vi "Main.vi"() -> ()   [LabVIEW 2021]
uses:
  controls/SynchroCheckCentral.ctl
  controls/SynchroCheckCentral_Info.ctl
  controls/SynchroCheckCentral_Data.ctl
  controls/3ph Phasor.ctl
  controls/Phasor.ctl
  controls/AFE_froming_Central.ctl
  controls/AFE_froming_Central_Info.ctl
  controls/AFE_froming_Central_Data.ctl
  controls/references.ctl
  controls/Connected_OPF.ctl
  controls/Connected_OPF_Info.ctl
  controls/Connected_OPF_Data.ctl
  controls/Optimal_slack_selection.ctl
  controls/Optimal_slack_selection_Info.ctl
  controls/Optimal_slack_selection_Data.ctl
  controls/PVemulator_Central.ctl
  controls/PVemulator_Central_Info.ctl
  controls/PVemulator_Central_Data.ctl
  controls/measurements.ctl
  controls/measurements_SC.ctl
  controls/SC_references.ctl
  controls/MeteoBoxCentral.ctl
  controls/MeteoBoxCentral_Info.ctl
  controls/MeteoBoxCentral_Data.ctl
  controls/Setpoints_CDA.ctl
  controls/Setpoints_CDA_ZENONE.ctl
  controls/SCADA_to_SM.ctl
  controls/SCADAOGCentral_Info.ctl
  controls/SCADA_to_SM_Data.ctl
  controls/State Machine.ctl
  <vilib>/Platform/TimedLoop/XDataNode/timing_clust.ctl
  <vilib>/Platform/TimedLoop/XDataNode/nitl_modes.ctl
  <vilib>/Platform/TimedLoop/XDataNode/wakeup.ctl
  controls/PV_facade_central.ctl
  controls/PV_facade_cental_Info.ctl
  controls/PV_facade_central_Data.ctl
  <vilib>/JDP Science/JSONtext/Next JSON Value.vi
  <vilib>/JDP Science/JSONtext/String Subset.vi
  <vilib>/JDP Science/JSONtext/Parsing/Advance past next JSON Value (inlined COPY).vi
  <vilib>/JDP Science/JSONtext/Parsing/Advance past whitespace.vi
  <vilib>/JDP Science/JSONtext/Parsing/Advance past String.vi
  <vilib>/JDP Science/JSONtext/Parsing/Advance past Number.vi
  <vilib>/JDP Science/JSONtext/Parsing/Advance past Line Ending.vi
  <vilib>/JDP Science/JSONtext/Parsing/Parse Full Path or Item Name.vi
  <vilib>/JDP Science/JSONtext/Parsing/Advance past Array.vi
  <vilib>/JDP Science/JSONtext/Parsing/Advance past Object.vi
  <vilib>/JDP Science/JSONtext/support/Error Cluster From Code.vi
  <vilib>/JDP Science/JSONtext/Offset/Find Item Locations by Path.vi
  <vilib>/Utility/file.llb/Read Delimited Spreadsheet (DBL).vi
  <vilib>/Platform/TimedLoop/XDataNode/XDataNode.xnode
  <vilib>/Platform/TimedLoop/XDataNode/XDNodeRunTimeDep.lvlib
  <vilib>/JDP Science/JSONtext/JSONtext.lvlib
  <userlib>/_OpenG.lib/boolean/boolean.llb/openg_boolean__ogtk.lvlib
panel:
  out "V_afe":dbl
  out "V_upstream":dbl
  out "V_control":dbl
  out "V control":cluster{dbl, "ROCOF [Hz/s]":dbl}(graph)
  in  "PI on V":bool
  in  "SCADA":T1={"Info"={"Resource"="MeteoBox", "Problem"=FALSE, "Timestamp"=0.0}, "Data"={"Voltage mag"=[], "Voltage angle"=[]}}
  out "SCADA data":bool
  in  "OUT":T4
  in  "SC_include":bool
  out "time connected":timestamp
  out "time island":timestamp
  out "P_bess_island":dbl
  out "P_bess_connected":dbl
  out "P_pv_facade":dbl
  in  "SOC":dbl=40.0
  in  "bias magnitude":dbl
  in  "IN Meteo":T6={"Info"={"Resource"="MeteoBox", "Problem"=FALSE, "Timestamp"=0.0}, "Data"={"GI"=0.0, "GHI"=0.0, "GVI"=0.0, "Tair"=0.0, "Tcell roof"=0.0, "Global_Total_Irr"=0.0, "Diffused_Irr"=0.0, "Tcell facade"=0.0, "PV_mpp"={"perun"=0.0, "solarmax"=0.0, "facade"=0.0, "emul4"=0.0, "emul5"=0.0, "emul6"=0.0, "emul7"=0.0}}}
  out "SC_soc":dbl
  out "delta angle":dbl
  in  "Send sp DC?":bool
  in  "Send sp AC?":bool
  out "Zenone_Q":dbl
  out "Zenone_P":dbl
  out "forming SC?":bool
  out "OUT PV+SC":T9={"Info"={"Resource"="Zenone", "Problem"=FALSE, "Timestamp"=0.0}, "Data"={"Status 1"=FALSE, "Status 2"=FALSE, "measurements"={"V_PV1"=0.0, "V_CAP1"=0.0, "V_PV2"=0.0, "V_CAP2"=0.0, "V_grid2"=0.0, "V_PV3"=0.0, "V_CAP3"=0.0, "V_grid3"=0.0, "V_PV4"=0.0, "V_CAP4"=0.0, "V_grid4"=0.0, "V_grid1"=0.0, "P1"=0.0, "P2"=0.0, "P3"=0.0, "P4"=0.0}, "Status 3"=FALSE, "Status 4"=FALSE, "measurements SC"={"V_SC"=0.0, "V_CAP"=0.0, "V_grid"=0.0, "P"=0.0, "SOC"=0.0}, "Status SC"=FALSE, "Forming/Following"=FALSE, "Start forming"=FALSE, "SC references"={"Vdc"=0.0, "Pdc"=0.0}, "Start following"=FALSE}}
  out "PV data":bool
  out "AFE data":bool
  out "synchro data":bool
  in  "IN PV+SC":T9={"Info"={"Resource"="Zenone", "Problem"=FALSE, "Timestamp"=0.0}, "Data"={"Status 1"=FALSE, "Status 2"=FALSE, "measurements"={"V_PV1"=0.0, "V_CAP1"=0.0, "V_PV2"=0.0, "V_CAP2"=0.0, "V_grid2"=0.0, "V_PV3"=0.0, "V_CAP3"=0.0, "V_grid3"=0.0, "V_PV4"=0.0, "V_CAP4"=0.0, "V_grid4"=0.0, "V_grid1"=0.0, "P1"=0.0, "P2"=0.0, "P3"=0.0, "P4"=0.0}, "Status 3"=FALSE, "Status 4"=FALSE, "measurements SC"={"V_SC"=0.0, "V_CAP"=0.0, "V_grid"=0.0, "P"=0.0, "SOC"=0.0}, "Status SC"=FALSE, "Forming/Following"=FALSE, "Start forming"=FALSE, "SC references"={"Vdc"=0.0, "Pdc"=0.0}, "Start following"=FALSE}}
  out "iOPF data":bool
  out "cOPF data":bool
  in  "slack":T15={"Info"={"Resource"="Zenone", "Problem"=FALSE, "Timestamp"=0.0}, "Data"={"Operation mode"="Grid connected", "Optimal slack"="AFE 1", "Time-To-Live"=0.0}}
  in  "IN AFE":T18={"Info"={"Resource"="Zenone", "Problem"=FALSE, "Timestamp"=0.0}, "Data"={"Start forming 1"=FALSE, "Forming/Following"=[], "Start forming 2"=FALSE, "measurements"={"Vdc1"=0.0, "P1"=0.0, "Vdc2"=0.0, "P2"=0.0, "Q2"=0.0, "Vdc3"=0.0, "P3"=0.0, "Q3"=0.0, "Vdc4"=0.0, "P4"=0.0, "Q4"=0.0, "Q1"=0.0}, "Status"=[], "references"={"Vdc1"=0.0, "Vdc2"=0.0, "Qac2"=0.0, "Vdc3"=0.0, "Qac3"=0.0, "Vdc4"=0.0, "Qac4"=0.0, "Qac1"=0.0, "V_arg2"=0.0, "V_abs2"=0.0, "V_abs1"=0.0, "V_arg1"=0.0, "freq1"=0.0, "freq2"=0.0}, "Start following 1"=FALSE, "Start following 2"=FALSE}}
  in  "IN cOPF":T22={"Info"={"Resource"="Zenone", "Problem"=0.0, "Timestamp"=0.0}, "Data"={"Operation_mode"="Grid connected", "solution_feasible"=0.0, "Optimal_slack"="AFE 1", "setpoints"=[], "upper_layer_grid_info"={"Frequency"=0.0, "Angle"=0.0, "Magnitude"=0.0}, "SC_soc"=0.0, "PV"={"perun"=0.0, "solarmax"=0.0, "facade"=0.0, "emul4"=0.0, "emul5"=0.0, "emul6"=0.0, "emul7"=0.0}, "P_pv_facade"=0.0}}
  in  "IN iOPF":T22={"Info"={"Resource"="Zenone", "Problem"=0.0, "Timestamp"=0.0}, "Data"={"Operation_mode"="Grid connected", "solution_feasible"=0.0, "Optimal_slack"="AFE 1", "setpoints"=[], "upper_layer_grid_info"={"Frequency"=0.0, "Angle"=0.0, "Magnitude"=0.0}, "SC_soc"=0.0, "PV"={"perun"=0.0, "solarmax"=0.0, "facade"=0.0, "emul4"=0.0, "emul5"=0.0, "emul6"=0.0, "emul7"=0.0}, "P_pv_facade"=0.0}}
  in  "IN synchro":T25={"Info"={"Resource"="SyncroCheck", "Problem"=FALSE, "Timestamp"=0.0}, "Data"={"close/open relay"=TRUE, "Operation mode"="Grid connected", "V_Downstream"={"Phase A"={"Frequency"=0.0, "Magnitude"=0.0, "Angle [Deg]"=0.0}, "Phase B"={"Frequency"=0.0, "Magnitude"=0.0, "Angle [Deg]"=0.0}, "Phase C"={"Frequency"=0.0, "Magnitude"=0.0, "Angle [Deg]"=0.0}, "Phase N"={"Frequency"=0.0, "Magnitude"=0.0, "Angle [Deg]"=0.0}}, "V_UpStream"={"Phase A"={"Frequency"=0.0, "Magnitude"=0.0, "Angle [Deg]"=0.0}, "Phase B"={"Frequency"=0.0, "Magnitude"=0.0, "Angle [Deg]"=0.0}, "Phase C"={"Frequency"=0.0, "Magnitude"=0.0, "Angle [Deg]"=0.0}, "Phase N"={"Frequency"=0.0, "Magnitude"=0.0, "Angle [Deg]"=0.0}}, "Synchronised?"=TRUE}}
  out "OUT iOPF":T22={"Info"={"Resource"="Zenone", "Problem"=0.0, "Timestamp"=0.0}, "Data"={"Operation_mode"="Grid connected", "solution_feasible"=0.0, "Optimal_slack"="AFE 1", "setpoints"=[], "upper_layer_grid_info"={"Frequency"=0.0, "Angle"=0.0, "Magnitude"=0.0}, "SC_soc"=0.0, "PV"={"perun"=0.0, "solarmax"=0.0, "facade"=0.0, "emul4"=0.0, "emul5"=0.0, "emul6"=0.0, "emul7"=0.0}, "P_pv_facade"=0.0}}
  out "OUT cOPF":T22={"Info"={"Resource"="Zenone", "Problem"=0.0, "Timestamp"=0.0}, "Data"={"Operation_mode"="Grid connected", "solution_feasible"=0.0, "Optimal_slack"="AFE 1", "setpoints"=[], "upper_layer_grid_info"={"Frequency"=0.0, "Angle"=0.0, "Magnitude"=0.0}, "SC_soc"=0.0, "PV"={"perun"=0.0, "solarmax"=0.0, "facade"=0.0, "emul4"=0.0, "emul5"=0.0, "emul6"=0.0, "emul7"=0.0}, "P_pv_facade"=0.0}}
  out "OUT AFE":T18={"Info"={"Resource"="Zenone", "Problem"=FALSE, "Timestamp"=0.0}, "Data"={"Start forming 1"=FALSE, "Forming/Following"=[], "Start forming 2"=FALSE, "measurements"={"Vdc1"=0.0, "P1"=0.0, "Vdc2"=0.0, "P2"=0.0, "Q2"=0.0, "Vdc3"=0.0, "P3"=0.0, "Q3"=0.0, "Vdc4"=0.0, "P4"=0.0, "Q4"=0.0, "Q1"=0.0}, "Status"=[], "references"={"Vdc1"=0.0, "Vdc2"=0.0, "Qac2"=0.0, "Vdc3"=0.0, "Qac3"=0.0, "Vdc4"=0.0, "Qac4"=0.0, "Qac1"=0.0, "V_arg2"=0.0, "V_abs2"=0.0, "V_abs1"=0.0, "V_arg1"=0.0, "freq1"=0.0, "freq2"=0.0}, "Start following 1"=FALSE, "Start following 2"=FALSE}}
  out "OUT Synchro":T25={"Info"={"Resource"="SyncroCheck", "Problem"=FALSE, "Timestamp"=0.0}, "Data"={"close/open relay"=TRUE, "Operation mode"="Grid connected", "V_Downstream"={"Phase A"={"Frequency"=0.0, "Magnitude"=0.0, "Angle [Deg]"=0.0}, "Phase B"={"Frequency"=0.0, "Magnitude"=0.0, "Angle [Deg]"=0.0}, "Phase C"={"Frequency"=0.0, "Magnitude"=0.0, "Angle [Deg]"=0.0}, "Phase N"={"Frequency"=0.0, "Magnitude"=0.0, "Angle [Deg]"=0.0}}, "V_UpStream"={"Phase A"={"Frequency"=0.0, "Magnitude"=0.0, "Angle [Deg]"=0.0}, "Phase B"={"Frequency"=0.0, "Magnitude"=0.0, "Angle [Deg]"=0.0}, "Phase C"={"Frequency"=0.0, "Magnitude"=0.0, "Angle [Deg]"=0.0}, "Phase N"={"Frequency"=0.0, "Magnitude"=0.0, "Angle [Deg]"=0.0}}, "Synchronised?"=TRUE}}
  out "Time-To-Live (minutes)":dbl=134.0
  out "setpoints":dbl[](array[numeric])
  in  "nb instances":i16=7
  out "optimal_slack":string(combo)="AFE 1"
  out "iOPF valid":bool
  out "forming AFE?":bool
  out "cOPF valid?":bool
  out "synchronised?":bool
  in  "to grid connection":bool
  in  "to prepare for grid connection":bool
  in  "to island":bool
  in  "Stop":bool
  in  "to prepare for island":bool
  # "Islanding Manoeuvre - State Machine"
  # "synchronised"
  # "opf connected OK"
  # "opf island OK"
  # "forming AFE?"
  # "forming SC?"
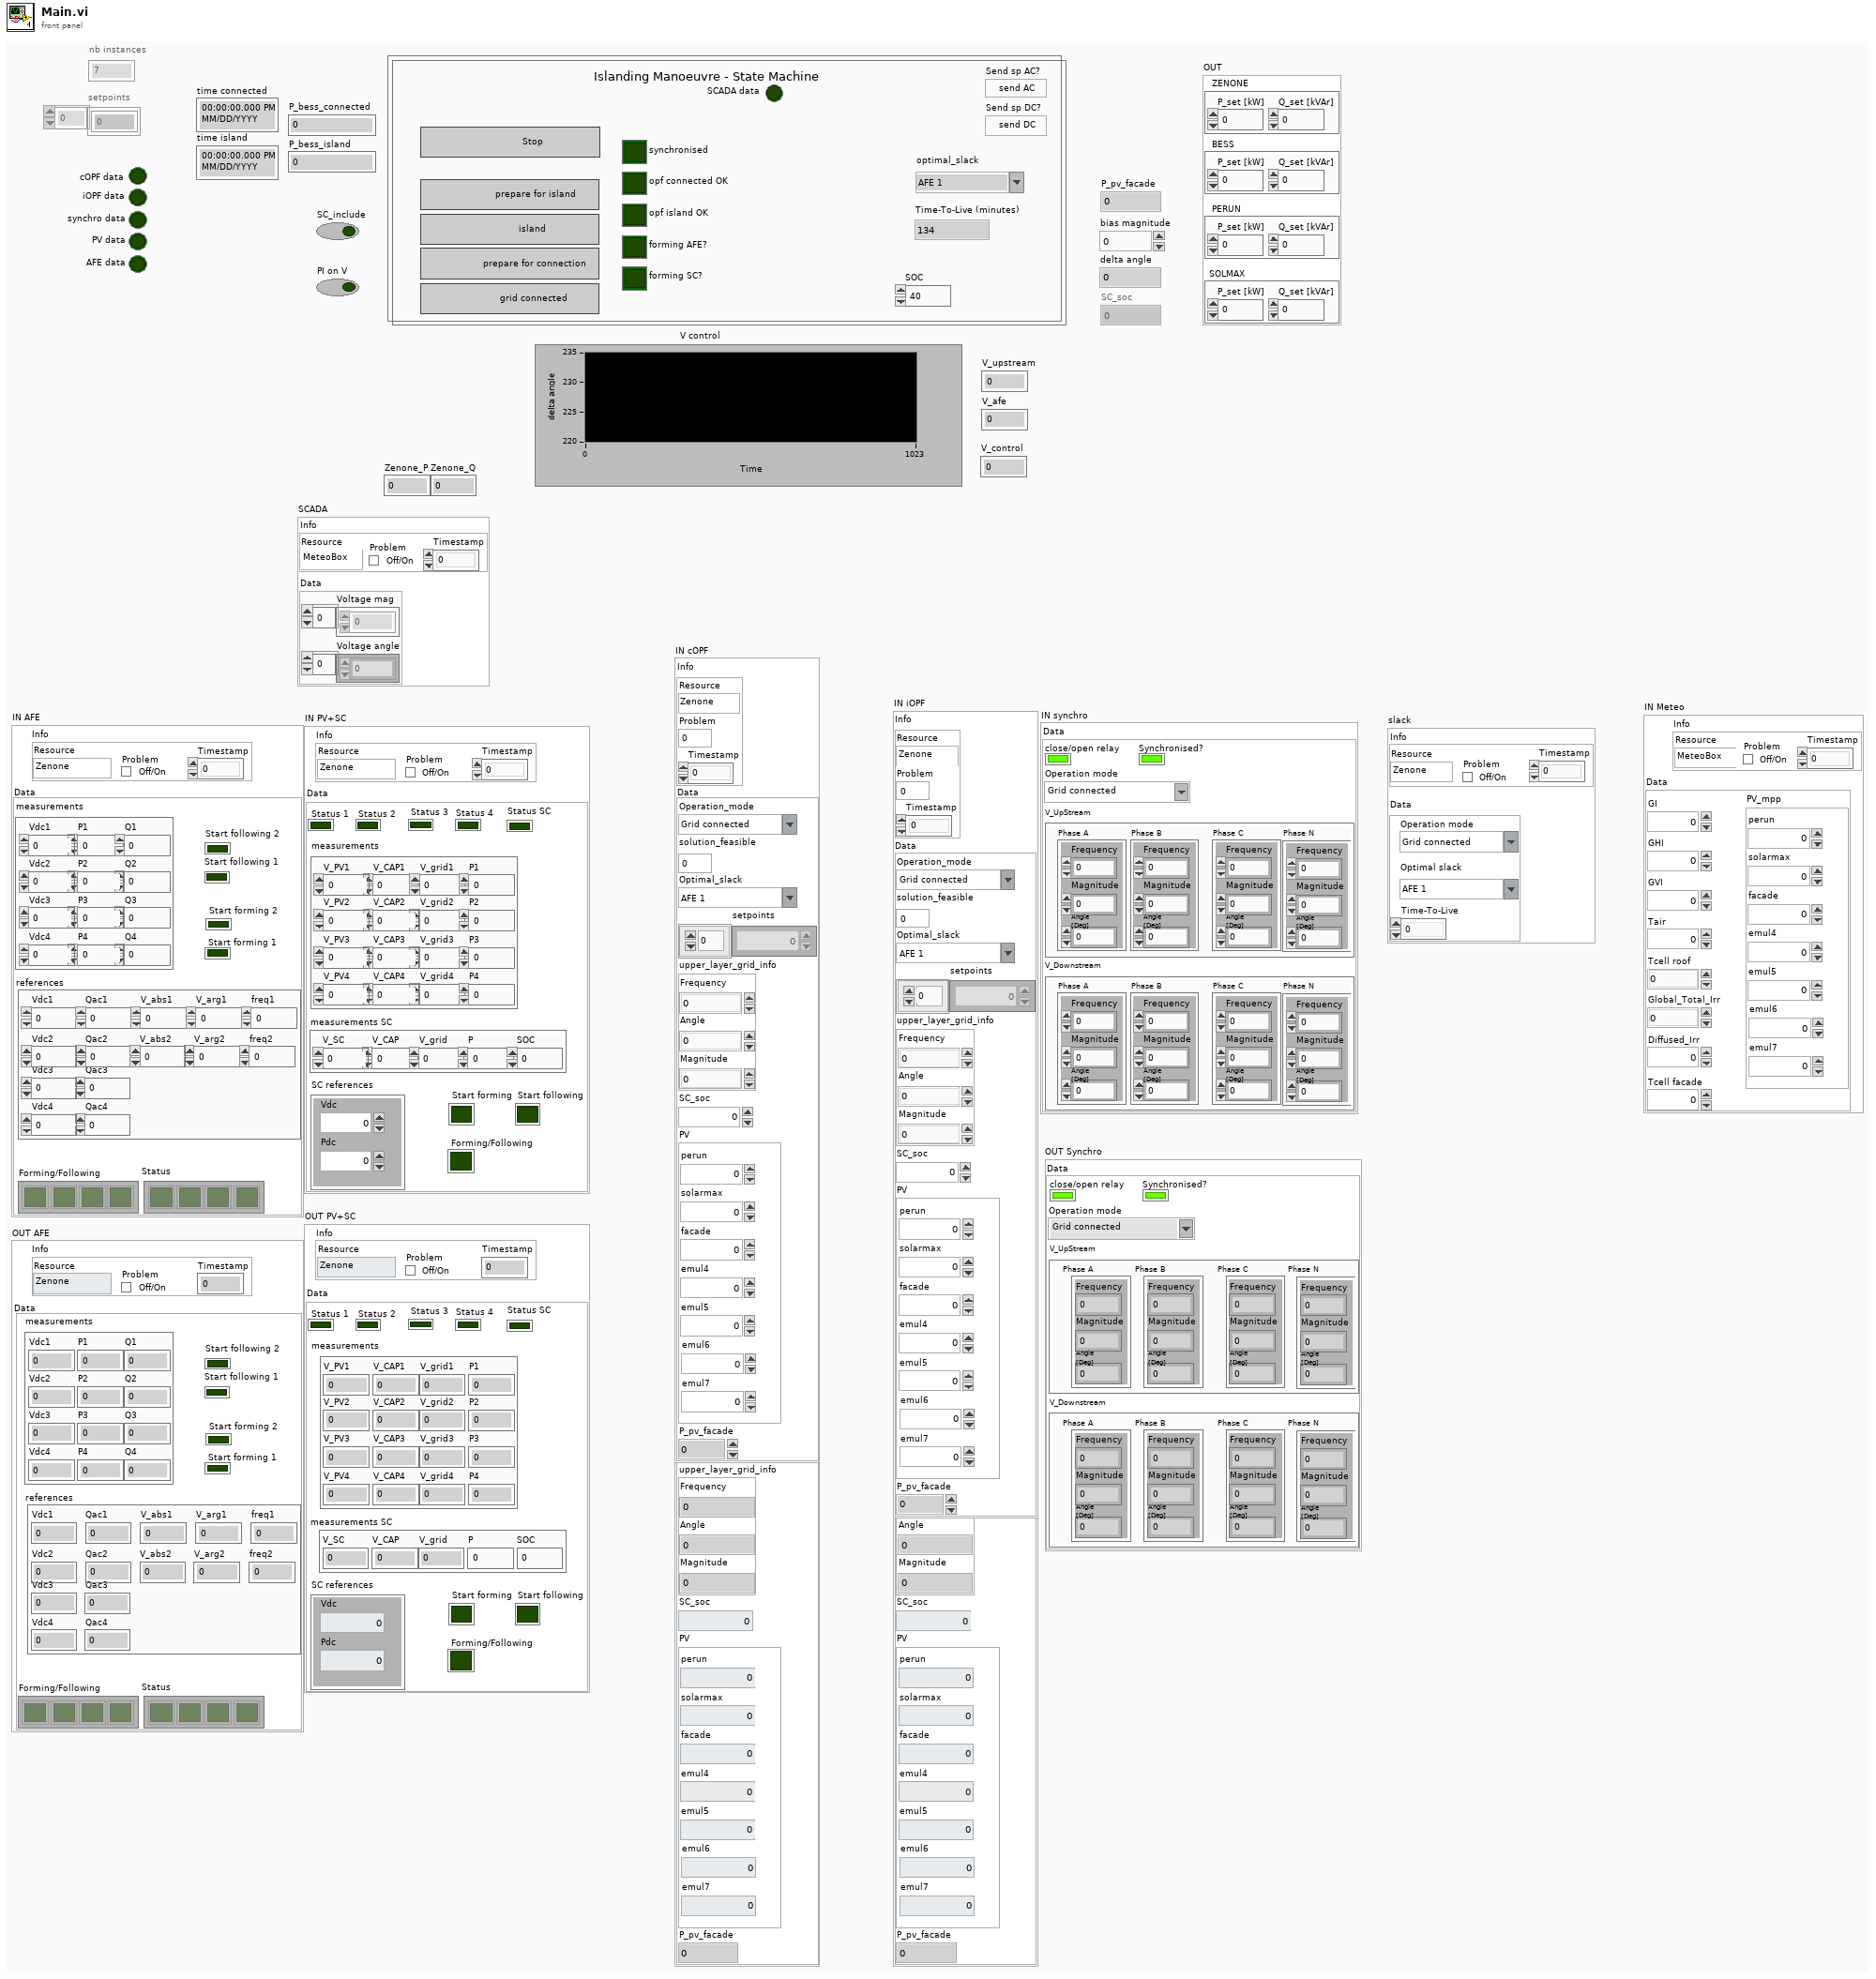
[diagram p1: front panel]
types:
  T1 = typedef "SCADA_to_SM.ctl" = cluster{"Info":T2, "Data":T3}
  T2 = typedef "SCADAOGCentral_Info.ctl" = cluster{"Resource":string, "Problem":bool, "Timestamp":dbl}
  T3 = typedef "SCADA_to_SM_Data.ctl" = cluster{"Voltage mag":dbl[], "Voltage angle":dbl[]}
  T4 = typedef "Setpoints_CDA.ctl" = cluster{"ZENONE":T5, "BESS":T5, "PERUN":T5, "SOLMAX":T5}
  T5 = typedef "Setpoints_CDA_ZENONE.ctl" = cluster{"P_set [kW]":dbl, "Q_set [kVAr]":dbl}
  T6 = typedef "MeteoBoxCentral.ctl" = cluster{"Info":T7, "Data":T8}
  T7 = typedef "MeteoBoxCentral_Info.ctl" = cluster{"Resource":string, "Problem":bool, "Timestamp":dbl}
  T8 = typedef "MeteoBoxCentral_Data.ctl" = cluster{"GI":dbl, "GHI":dbl, "GVI":dbl, "Tair":dbl, "Tcell roof":dbl, "Global_Total_Irr":dbl, "Diffused_Irr":dbl, "Tcell facade":dbl, "PV_mpp":cluster{"perun":dbl, "solarmax":dbl, "facade":dbl, "emul4":dbl, "emul5":dbl, "emul6":dbl, "emul7":dbl}}
  T9 = typedef "PVemulator_Central.ctl" = cluster{"Info":T10, "Data":T11}
  T10 = typedef "PVemulator_Central_Info.ctl" = cluster{"Resource":string, "Problem":bool, "Timestamp":dbl}
  T11 = typedef "PVemulator_Central_Data.ctl" = cluster{"Status 1":bool, "Status 2":bool, "measurements":T12, "Status 3":bool, "Status 4":bool, "measurements SC":T13, "Status SC":bool, "Forming/Following":bool, "Start forming":bool, "SC references":T14, "Start following":bool}
  T12 = typedef "measurements.ctl" = cluster{"V_PV1":dbl, "V_CAP1":dbl, "V_PV2":dbl, "V_CAP2":dbl, "V_grid2":dbl, "V_PV3":dbl, "V_CAP3":dbl, "V_grid3":dbl, "V_PV4":dbl, "V_CAP4":dbl, "V_grid4":dbl, "V_grid1":dbl, "P1":dbl, "P2":dbl, "P3":dbl, "P4":dbl}
  T13 = typedef "measurements_SC.ctl" = cluster{"V_SC":dbl, "V_CAP":dbl, "V_grid":dbl, "P":dbl, "SOC":dbl}
  T14 = typedef "SC_references.ctl" = cluster{"Vdc":dbl, "Pdc":dbl}
  T15 = typedef "Optimal_slack_selection.ctl" = cluster{"Info":T16, "Data":T17}
  T16 = typedef "Optimal_slack_selection_Info.ctl" = cluster{"Resource":string, "Problem":bool, "Timestamp":dbl}
  T17 = typedef "Optimal_slack_selection_Data.ctl" = cluster{"Operation mode":string, "Optimal slack":string, "Time-To-Live":dbl}
  T18 = typedef "AFE_froming_Central.ctl" = cluster{"Info":T19, "Data":T20}
  T19 = typedef "AFE_froming_Central_Info.ctl" = cluster{"Resource":string, "Problem":bool, "Timestamp":dbl}
  T20 = typedef "AFE_froming_Central_Data.ctl" = cluster{"Start forming 1":bool, "Forming/Following":bool[], "Start forming 2":bool, "measurements":cluster{"Vdc1":dbl, "P1":dbl, "Vdc2":dbl, "P2":dbl, "Q2":dbl, "Vdc3":dbl, "P3":dbl, "Q3":dbl, "Vdc4":dbl, "P4":dbl, "Q4":dbl, "Q1":dbl}, "Status":bool[], "references":T21, "Start following 1":bool, "Start following 2":bool}
  T21 = typedef "references.ctl" = cluster{"Vdc1":dbl, "Vdc2":dbl, "Qac2":dbl, "Vdc3":dbl, "Qac3":dbl, "Vdc4":dbl, "Qac4":dbl, "Qac1":dbl, "V_arg2":dbl, "V_abs2":dbl, "V_abs1":dbl, "V_arg1":dbl, "freq1":dbl, "freq2":dbl}
  T22 = typedef "Connected_OPF.ctl" = cluster{"Info":T23, "Data":T24}
  T23 = typedef "Connected_OPF_Info.ctl" = cluster{"Resource":string, "Problem":dbl, "Timestamp":dbl}
  T24 = typedef "Connected_OPF_Data.ctl" = cluster{"Operation_mode":string, "solution_feasible":dbl, "Optimal_slack":string, "setpoints":dbl[], "upper_layer_grid_info":cluster{"Frequency":dbl, "Angle":dbl, "Magnitude":dbl}, "SC_soc":dbl, "PV":cluster{"perun":dbl, "solarmax":dbl, "facade":dbl, "emul4":dbl, "emul5":dbl, "emul6":dbl, "emul7":dbl}, "P_pv_facade":dbl}
  T25 = typedef "SynchroCheckCentral.ctl" = cluster{"Info":T26, "Data":T27}
  T26 = typedef "SynchroCheckCentral_Info.ctl" = cluster{"Resource":string, "Problem":bool, "Timestamp":dbl}
  T27 = typedef "SynchroCheckCentral_Data.ctl" = cluster{"close/open relay":bool, "Operation mode":string, "V_Downstream":T28, "V_UpStream":T28, "Synchronised?":bool}
  T28 = typedef "3ph Phasor.ctl" = cluster{"Phase A":T29, "Phase B":T29, "Phase C":T29, "Phase N":T29}
  T29 = typedef "Phasor.ctl" = cluster{"Frequency":dbl, "Magnitude":dbl, "Angle [Deg]":dbl}
  T30 = typedef "State Machine.ctl" = enum16{"Grid connected", "Prepare for island", "Forming but connected", "Island", "Prepare for connection"}
  T31 = typedef "PV_facade_central.ctl" = cluster{"Info":T32, "Data":T33}
  T32 = typedef "PV_facade_cental_Info.ctl" = cluster{"Resource":string, "Problem":bool, "Timestamp":dbl}
  T33 = typedef "PV_facade_central_Data.ctl" = cluster{"P":dbl, "Q":dbl, "Pset":dbl, "Qset":dbl}
  T34 = typedef "XDNodeRunTimeDep.lvlib/timing_clust.ctl" = cluster{"Expected End [f-1]":u64, "Actual End [f-1]":u64, "Finished Late? [f-1]":bool, "Expected End [i-1]":u64, "Actual End [i-1]":u64, "Finished Late? [i-1]":bool, "Expected Start [i]":u64, "Actual Start [i]":u64, "Expected Start [f]":u64, "Actual Start [f]":u64, "Source Name":string, "Structure Name":string, "Period":i64, "Deadline":i64, "Offset":i64, "Start":i64, "Priority":i32, "Timeout":i32, "Mode":T35, "Wakeup Reason":T36, "Error":errorcluster, "Source Type":string, "Secondary Source Type":string, "Global End Time":u64, "Global Start Time":u64, "Frame Duration":u64, "Iteration Duration":u64, "Assigned CPU":i32, "I/O Scan Engine Mode":u32}
  T35 = typedef "XDNodeRunTimeDep.lvlib/nitl_modes.ctl" = enum32{"No Change", "Process missed periods, maintain original phase", "Discard missed periods, maintain original phase", "Process missed periods, ignore original phase", "Discard missed periods, ignore original phase"}
  T36 = typedef "XDNodeRunTimeDep.lvlib/wakeup.ctl" = enum32{"Normal", "Aborted", "Asynchronous wakeup", "Timing source error", "Timed loop error", "Timeout"}
  T37 = cluster{"Frequency":dbl, "Angle":dbl, "Magnitude":dbl}
  T38 = cluster{"perun":dbl, "solarmax":dbl, "facade":dbl, "emul4":dbl, "emul5":dbl, "emul6":dbl, "emul7":dbl}
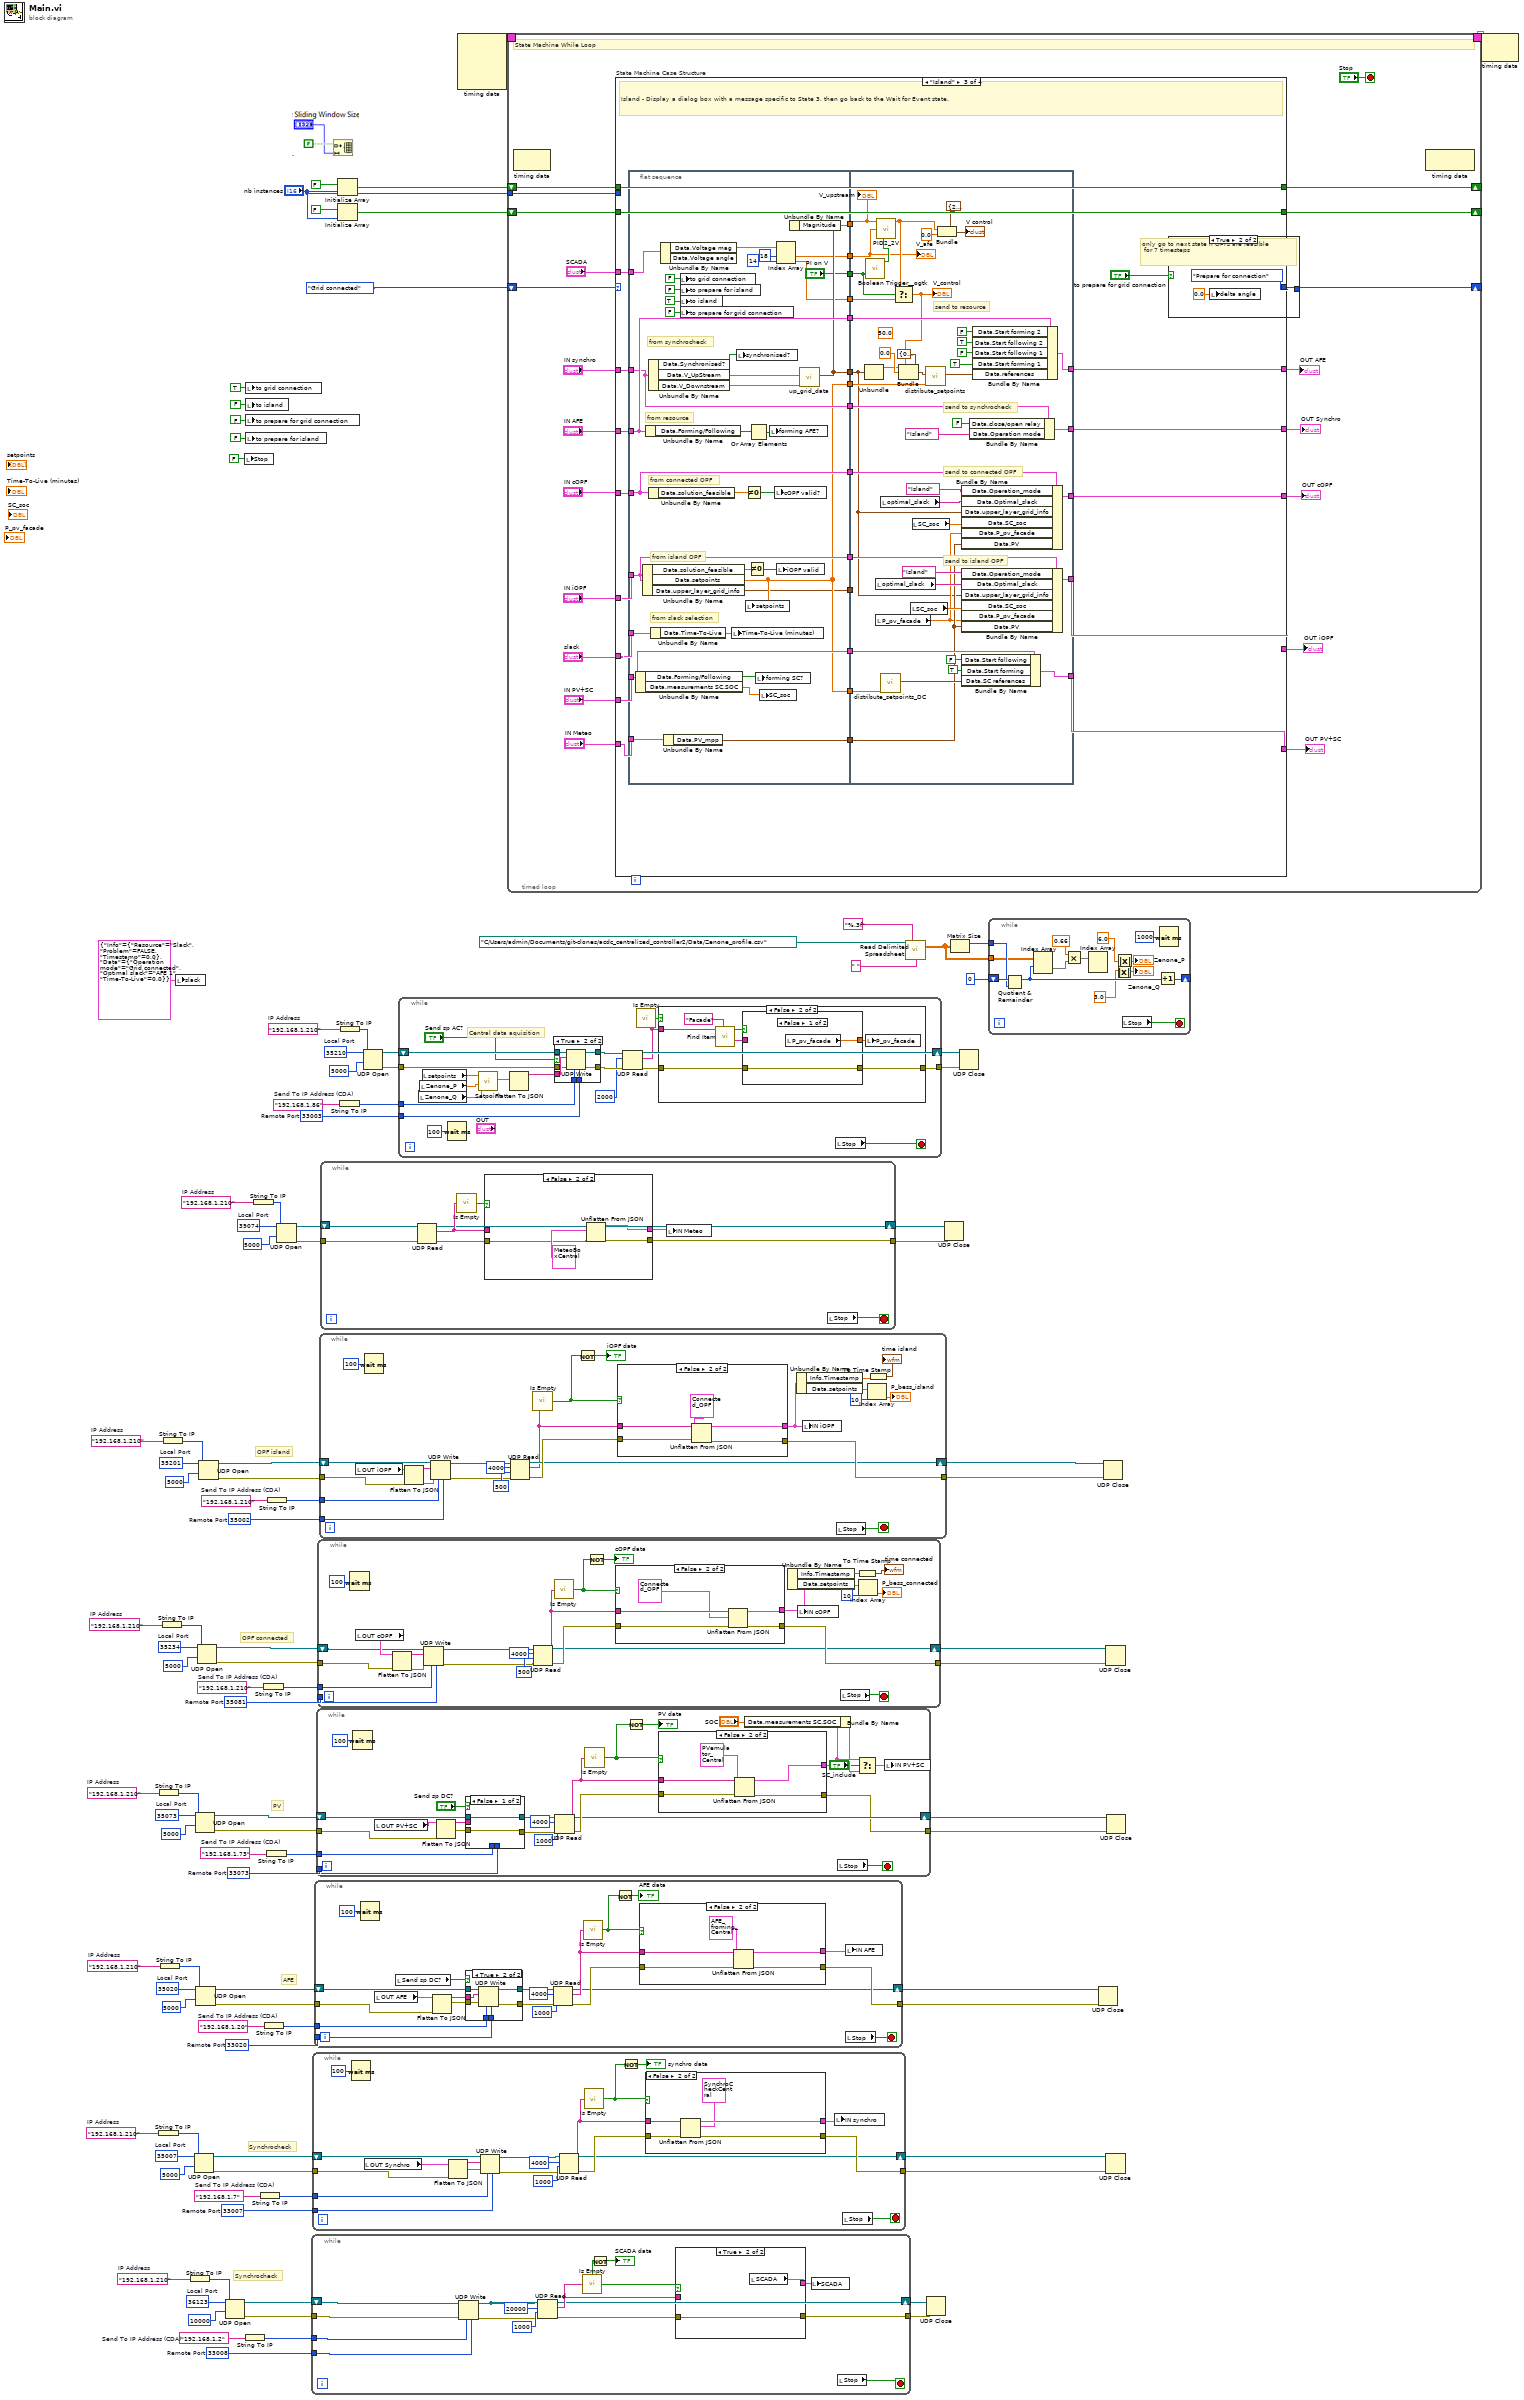
[diagram p0: block diagram]
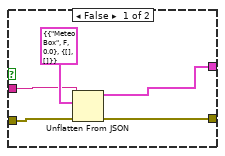
[diagram p2: hidden frame]
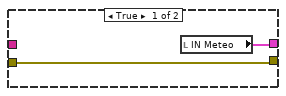
[diagram p3: hidden frame]
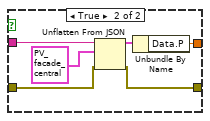
[diagram p5: hidden frame]
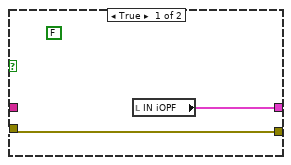
[diagram p7: hidden frame]
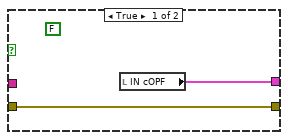
[diagram p8: hidden frame]
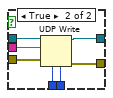
[diagram p9: hidden frame]
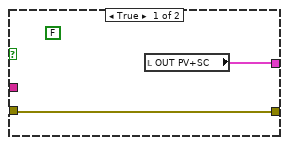
[diagram p10: hidden frame]
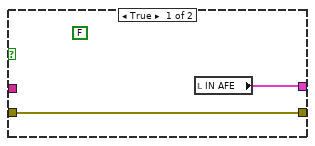
[diagram p12: hidden frame]
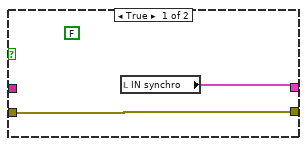
[diagram p13: hidden frame]
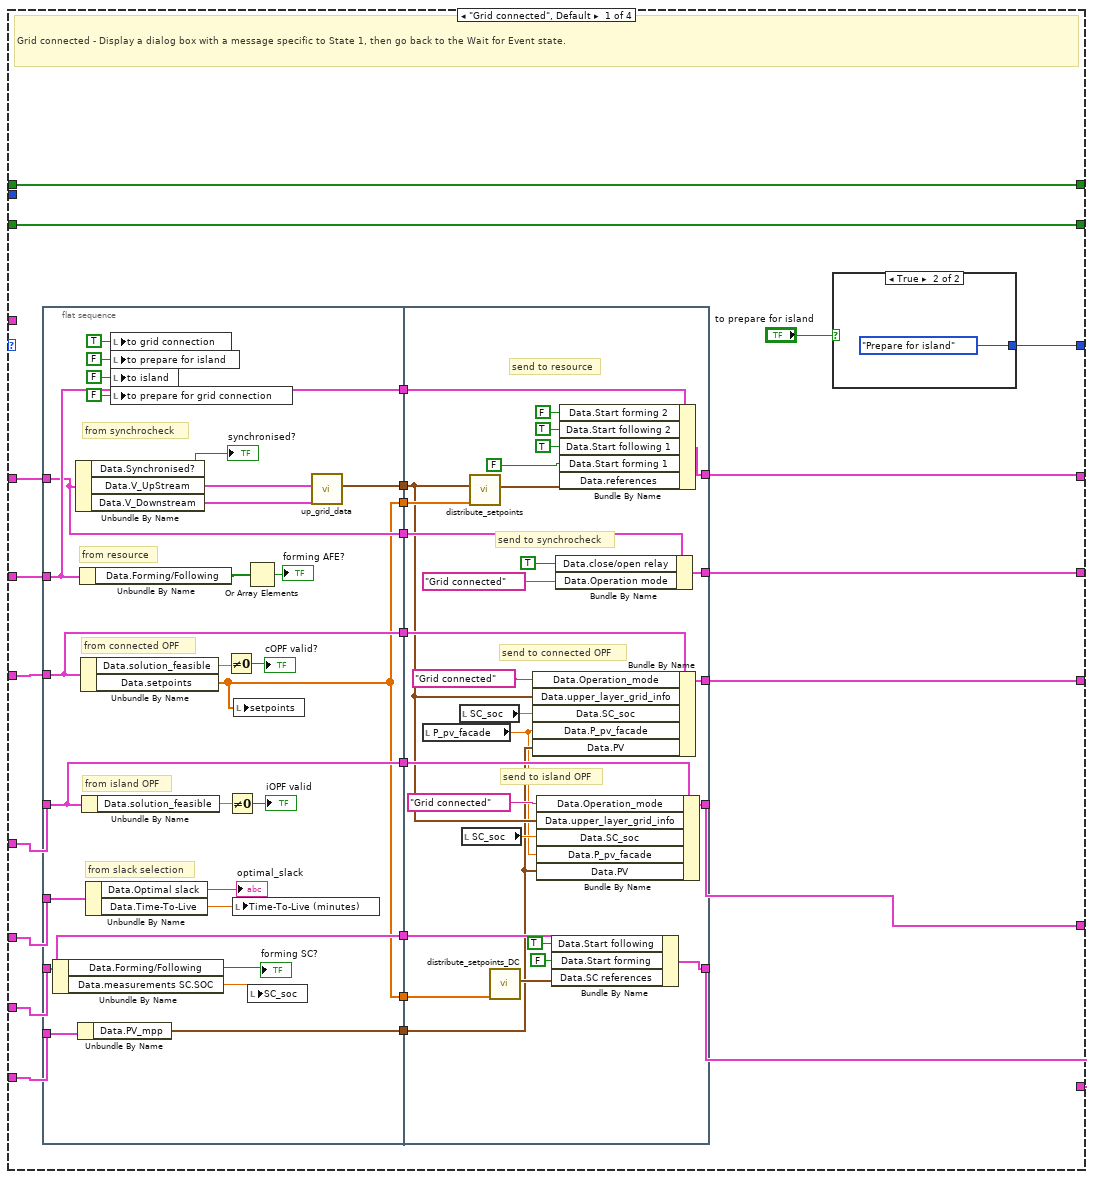
[diagram p14: hidden frame]
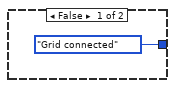
[diagram p15: hidden frame]
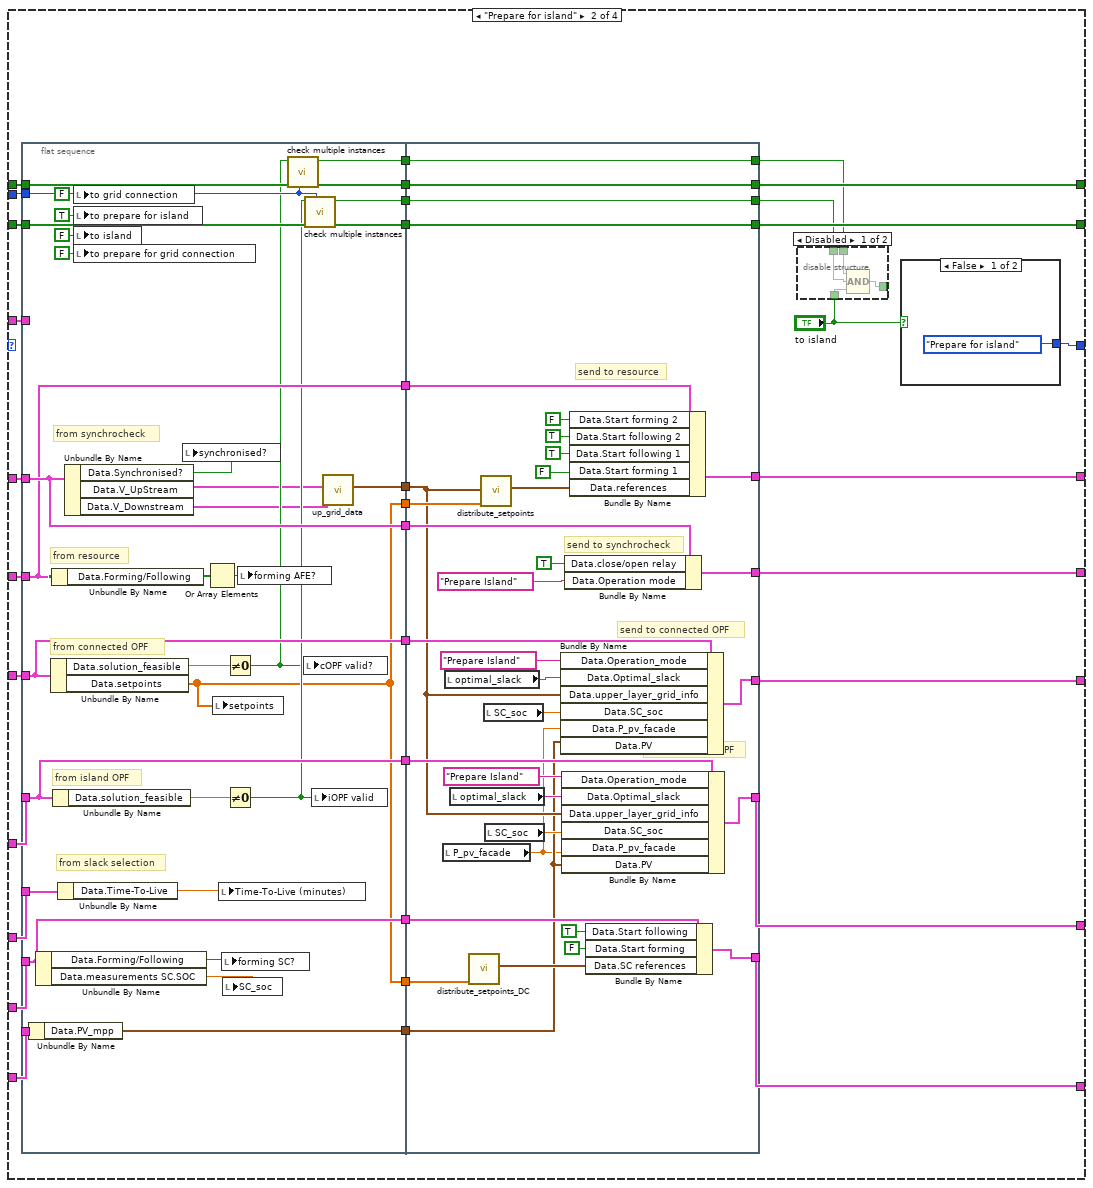
[diagram p16: hidden frame]
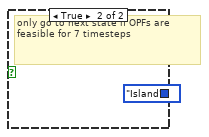
[diagram p18: hidden frame]
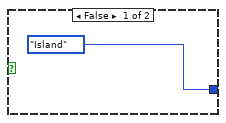
[diagram p19: hidden frame]
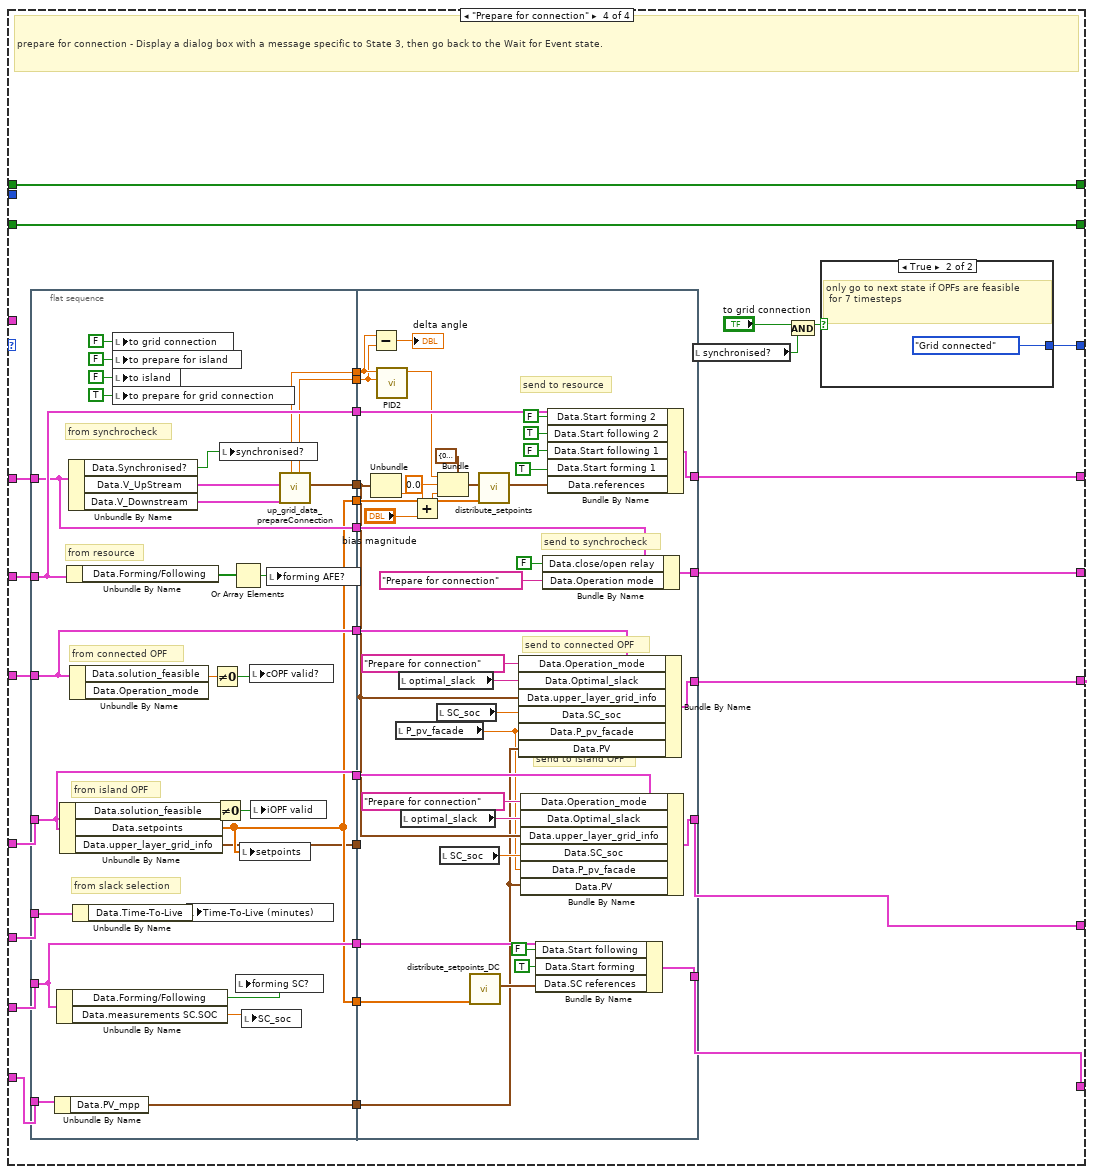
[diagram p20: hidden frame]
diagram:
  w3 = u16 33008  # Remote Port
  w7 = "192.168.1.2"  # Send To IP Address (CDA)
  w8 = u16 36123  # Local Port
  w10 = "192.168.1.210"  # IP Address
  w17 = u16 39074  # Local Port
  w19 = "192.168.1.210"  # IP Address
  w28 = u16 33003  # Remote Port
  w30 = "192.168.1.86"  # Send To IP Address (CDA)
  w32 = u16 35210  # Local Port
  w34 = "192.168.1.210"  # IP Address
  w57 = u16 33073  # Remote Port
  w58 = "192.168.1.73"  # Send To IP Address (CDA)
  w53 = u16 33020  # Remote Port
  w61 = "192.168.1.20"  # Send To IP Address (CDA)
  w48 = u16 33007  # Remote Port
  w62 = "192.168.1.7"  # Send To IP Address (CDA)
  w63 = u16 35007  # Local Port
  w65 = "192.168.1.210"  # IP Address
  w67 = u16 35020  # Local Port
  w69 = "192.168.1.210"  # IP Address
  w71 = u16 35073  # Local Port
  w73 = "192.168.1.210"  # IP Address
  w76 = u16 35002  # Remote Port
  w77 = "192.168.1.210"  # Send To IP Address (CDA)
  w78 = u16 35081  # Remote Port
  w80 = "192.168.1.210"  # Send To IP Address (CDA)
  w87 = u16 35234  # Local Port
  w89 = "192.168.1.210"  # IP Address
  w93 = u16 35201  # Local Port
  w95 = "192.168.1.210"  # IP Address
  # "Synchrocheck"
  # "Synchrocheck"
  # "AFE"
  # "PV"
  # "OPF connected"
  # "OPF island"
  n1 = String To IP(1:w65) -> (0:w66:u32)
  n2 = String To IP(1:w73) -> (0:w74:u32)
  n3 = String To IP(1:w69) -> (0:w70:u32)
  n4 = String To IP(1:w89) -> (0:w90:u32)
  n5 = String To IP(1:w95) -> (0:w96:u32)
  n6 = local write "slack"(T15 {"Info"={"Resource"="Slack", "Problem"=FALSE, "Timestamp"=0.0}, "Data"={"Operation mode"="Grid connected", "Optimal slack"="AFE 1", "Time-To-Live"=0.0}} ("slack")) -> ()
  n7 = String To IP(1:w10) -> (0:w11:u32)
  n8 = UDP Open(7:w66, 9:5000 ("timeout ms (25000)"), 11:w63) -> (port=w51:refnum<k16>, 0:w50:errorcluster)  [unwired: 2 in, 1 out]
  n9 = UDP Open(7:w74, 9:5000 ("timeout ms (25000)"), 11:w71) -> (port=w60:refnum<k16>, 0:w59:errorcluster)  [unwired: 2 in, 1 out]
  n10 = UDP Open(7:w70, 9:5000 ("timeout ms (25000)"), 11:w67) -> (port=w55:refnum<k16>, 0:w54:errorcluster)  [unwired: 2 in, 1 out]
  n11 = UDP Open(7:w90, 9:5000 ("timeout ms (25000)"), 11:w87) -> (port=w86:refnum<k16>, 0:w85:errorcluster)  [unwired: 2 in, 1 out]
  n12 = UDP Open(7:w96, 9:5000 ("timeout ms (25000)"), 11:w93) -> (port=w92:refnum<k16>, 0:w91:errorcluster)  [unwired: 2 in, 1 out]
  n13 = UDP Open(7:w11, 9:10000 ("timeout ms (25000)"), 11:w8) -> (port=w6:refnum<k16>, 0:w5:errorcluster)  [unwired: 2 in, 1 out]
  n14 = local write "Stop"(FALSE ("Stop")) -> ()
  n15 = local write "to grid connection"(TRUE ("to grid connection")) -> ()
  n16 = local write "to island"(FALSE ("to island")) -> ()
  n17 = local write "to prepare for grid connection"(FALSE ("to prepare for grid connection")) -> ()
  n18 = local write "to prepare for island"(FALSE ("to prepare for island")) -> ()
  n19 = String To IP(1:w7) -> (0:w4:u32)
  n20 = String To IP(1:w19) -> (0:w20:u32)
  n21 = String To IP(1:w62) -> (0:w49:u32)
  n22 = String To IP(1:w80) -> (0:w79:u32)
  n23 = String To IP(1:w61) -> (0:w52:u32)
  n24 = String To IP(1:w58) -> (0:w56:u32)
  n25 = String To IP(1:w77) -> (0:w75:u32)
  n26 = UDP Open(7:w20, 9:5000 ("timeout ms (25000)"), 11:w17) -> (port=w16:refnum<k16>, 0:w15:errorcluster)  [unwired: 2 in, 1 out]
  n27 = while {
    tunnel: w5 -> [w114]
    tunnel: w4 -> [w113]
    tunnel: w3 -> [w112]
    shift-right: [w109] -> w2
    shift-left: w6 -> [w115]
    tunnel: [w107] -> w1
    stop <- w120 stop-if-true
    n28 = UDP Write(address=w113, port or service name=w112, connection ID=w115, 8:w114) -> (error out=w117:errorcluster, 3:w109:refnum<k16>)  [unwired: 2 in]
    n29 = UDP Read(connection ID=w109, max size (548)=20000, timeout ms (25000)=1000, 8:w117) -> (data out=w110:string, error out=w108:errorcluster)  [unwired: 3 out]
    n30 = call <vilib>:"Is Empty.vi"("JSON"=w110) -> ("Empty"=w111:bool)  [unwired: 4 in]
    n31 = Not(x=w111) -> (.not. x?=→"SCADA data":bool)
    n32 = case shown="True" w111 {
      tunnel: w110 -> [w124 _]
      tunnel: w108 -> [w123 w126]
      tunnel: [w122 w126] -> w107
      tunnel: [w121 w127] -> w106
      frame False {
        n33 = Unflatten From JSON(JSON string=w124, type and defaults=T1 {"Info"={"Resource"="MeteoBox", "Problem"=FALSE, "Timestamp"=0.0}, "Data"={"Voltage mag"=[], "Voltage angle"=[]}} ("Cluster"), error in (no error)=w123) -> (value=w121:T1, error out=w122:errorcluster)  [unwired: 4 in]
      }
      frame True {
        n34 = local read "SCADA"() -> (w127:T1)
      }
    }
    n35 = local write "SCADA"(w106) -> ()
    n36 = local read "Stop"() -> (w120:bool)
  }
  n37 = while {
    tunnel: w49 -> [w147]
    tunnel: w48 -> [w146]
    shift-right: [w132] -> w47
    shift-left: w51 -> [w130]
    tunnel: w50 -> [w128]
    tunnel: [w133] -> w46
    stop <- w135 stop-if-true
    n38 = Wait (ms)(milliseconds to wait=u32 100) -> ()  [unwired: 1 out]
    n39 = local read "OUT Synchro"() -> (w140:T25)
    n40 = Flatten To JSON(anything=w140, error in (no error)=w128) -> (JSON string=w134:string, 11:w141:errorcluster)  [unwired: 1 in]
    n41 = UDP Write(address=w147, port or service name=w146, connection ID=w130, data in=w134, 8:w141) -> (error out=w129:errorcluster, 3:w131:refnum<k16>)  [unwired: 1 in]
    n42 = UDP Read(connection ID=w131, max size (548)=4000, timeout ms (25000)=1000, 8:w129) -> (data out=w145:string, error out=w137:errorcluster, 3:w132:refnum<k16>)  [unwired: 2 out]
    n43 = call <vilib>:"Is Empty.vi"("JSON"=w145) -> ("Empty"=w138:bool)  [unwired: 4 in]
    n44 = Not(x=w138) -> (.not. x?=→"synchro data":bool)
    n45 = case shown="False" w138 {
      tunnel: w137 -> [w149 w151]
      tunnel: [w148 w154] -> w142
      tunnel: w145 -> [_ w150]
      tunnel: [w149 w153] -> w133
      frame True {
        (unwired) FALSE ("Found")
        n46 = local read "IN synchro"() -> (w148:T25)
      }
      frame False {
        n47 = Unflatten From JSON(JSON string=w150, type and defaults=T25 {"Info"={"Resource"="SyncroCheck", "Problem"=FALSE, "Timestamp"=0.0}, "Data"={"close/open relay"=TRUE, "Operation mode"="Grid connected", "V_Downstream"={"Phase A"={"Frequency"=0.0, "Magnitude"=0.0, "Angle [Deg]"=0.0}, "Phase B"={"Frequency"=0.0, "Magnitude"=0.0, "Angle [Deg]"=0.0}, "Phase C"={"Frequency"=0.0, "Magnitude"=0.0, "Angle [Deg]"=0.0}, "Phase N"={"Frequency"=0.0, "Magnitude"=0.0, "Angle [Deg]"=0.0}}, "V_UpStream"={"Phase A"={"Frequency"=0.0, "Magnitude"=0.0, "Angle [Deg]"=0.0}, "Phase B"={"Frequency"=0.0, "Magnitude"=0.0, "Angle [Deg]"=0.0}, "Phase C"={"Frequency"=0.0, "Magnitude"=0.0, "Angle [Deg]"=0.0}, "Phase N"={"Frequency"=0.0, "Magnitude"=0.0, "Angle [Deg]"=0.0}}, "Synchronised?"=TRUE}} ("IN synchro"), error in (no error)=w151) -> (value=w154:T25, error out=w153:errorcluster)  [unwired: 4 in]
      }
    }
    n48 = local write "IN synchro"(w142) -> ()
    n49 = local read "Stop"() -> (w135:bool)
  }
  n50 = while {
    tunnel: w53 -> [w175]
    tunnel: w52 -> [w174]
    shift-right: [w158] -> w43
    shift-left: w55 -> [w160]
    tunnel: w54 -> [w162]
    tunnel: [w164] -> w42
    stop <- w166 stop-if-true
    n51 = Wait (ms)(milliseconds to wait=u32 100) -> ()  [unwired: 1 out]
    n52 = local read "OUT AFE"() -> (w157:T18)
    n53 = local read "Send sp DC?"() -> (w155:bool)
    n54 = Flatten To JSON(anything=w157, error in (no error)=w162) -> (JSON string=w165:string, 11:w170:errorcluster)  [unwired: 1 in]
    n55 = case shown="True" w155 {
      tunnel: w175 -> [_ w184]
      tunnel: w174 -> [_ w183]
      tunnel: w170 -> [w176 w182]
      tunnel: w165 -> [_ w181]
      tunnel: [w176 w180] -> w163
      tunnel: [w177 w179] -> w161
      tunnel: w160 -> [w177 w178]
      frame False {
      }
      frame True {
        n56 = UDP Write(address=w183, port or service name=w184, connection ID=w178, data in=w181, 8:w182) -> (error out=w180:errorcluster, 3:w179:refnum<k16>)  [unwired: 1 in]
      }
    }
    n57 = UDP Read(connection ID=w161, max size (548)=4000, timeout ms (25000)=1000, 8:w163) -> (data out=w159:string, error out=w171:errorcluster, 3:w158:refnum<k16>)  [unwired: 2 out]
    n58 = call <vilib>:"Is Empty.vi"("JSON"=w159) -> ("Empty"=w168:bool)  [unwired: 4 in]
    n59 = Not(x=w168) -> (.not. x?=→"AFE data":bool)
    n60 = case shown="False" w168 {
      tunnel: w171 -> [w186 w190]
      tunnel: [w185 w188] -> w156
      tunnel: w159 -> [_ w189]
      tunnel: [w186 w191] -> w164
      frame True {
        (unwired) FALSE ("Found")
        n61 = local read "IN AFE"() -> (w185:T18)
      }
      frame False {
        n62 = Unflatten From JSON(JSON string=w189, type and defaults=T18 {"Info"={"Resource"="Zenone", "Problem"=FALSE, "Timestamp"=0.0}, "Data"={"Start forming 1"=FALSE, "Forming/Following"=[], "Start forming 2"=FALSE, "measurements"={"Vdc1"=0.0, "P1"=0.0, "Vdc2"=0.0, "P2"=0.0, "Q2"=0.0, "Vdc3"=0.0, "P3"=0.0, "Q3"=0.0, "Vdc4"=0.0, "P4"=0.0, "Q4"=0.0, "Q1"=0.0}, "Status"=[], "references"={"Vdc1"=0.0, "Vdc2"=0.0, "Qac2"=0.0, "Vdc3"=0.0, "Qac3"=0.0, "Vdc4"=0.0, "Qac4"=0.0, "Qac1"=0.0, "V_arg2"=0.0, "V_abs2"=0.0, "V_abs1"=0.0, "V_arg1"=0.0, "freq1"=0.0, "freq2"=0.0}, "Start following 1"=FALSE, "Start following 2"=FALSE}} ("IN AFE"), error in (no error)=w190) -> (value=w188:T18, error out=w191:errorcluster)  [unwired: 4 in]
      }
    }
    n63 = local write "IN AFE"(w156) -> ()
    n64 = local read "Stop"() -> (w166:bool)
  }
  n65 = while {
    tunnel: w57 -> [w216]
    tunnel: w56 -> [w198]
    shift-right: [w203] -> w45
    shift-left: w60 -> [w206]
    tunnel: w59 -> [w202]
    tunnel: [w200] -> w44
    stop <- w207 stop-if-true
    n66 = Wait (ms)(milliseconds to wait=u32 100) -> ()  [unwired: 1 out]
    n67 = local read "OUT PV+SC"() -> (w199:T9)
    n68 = Flatten To JSON(anything=w199, error in (no error)=w202) -> (JSON string=w209:string, 11:w212:errorcluster)  [unwired: 1 in]
    n69 = case shown="False" "Send sp DC?" {
      tunnel: w216 -> [_ w225]
      tunnel: w198 -> [_ w224]
      tunnel: w212 -> [w217 w223]
      tunnel: w209 -> [_ w222]
      tunnel: w206 -> [w218 w221]
      tunnel: [w218 w220] -> w204
      tunnel: [w217 w219] -> w201
      frame False {
      }
      frame True {
        n70 = UDP Write(address=w224, port or service name=w225, connection ID=w221, data in=w222, 8:w223) -> (error out=w219:errorcluster, 3:w220:refnum<k16>)  [unwired: 1 in]
      }
    }
    n71 = UDP Read(connection ID=w204, max size (548)=4000, timeout ms (25000)=1000, 8:w201) -> (data out=w215:string, error out=w213:errorcluster, 3:w203:refnum<k16>)  [unwired: 2 out]
    n72 = call <vilib>:"Is Empty.vi"("JSON"=w215) -> ("Empty"=w210:bool)  [unwired: 4 in]
    n73 = Not(x=w210) -> (.not. x?=→"PV data":bool)
    n74 = case shown="False" w210 {
      tunnel: w213 -> [w227 w230]
      tunnel: [w226 w232] -> w194
      tunnel: w215 -> [_ w229]
      tunnel: [w227 w231] -> w200
      frame True {
        (unwired) FALSE ("Found")
        n75 = local read "OUT PV+SC"() -> (w226:T9)
      }
      frame False {
        n76 = Unflatten From JSON(JSON string=w229, type and defaults=T9 {"Info"={"Resource"="Zenone", "Problem"=FALSE, "Timestamp"=0.0}, "Data"={"Status 1"=FALSE, "Status 2"=FALSE, "measurements"={"V_PV1"=0.0, "V_CAP1"=0.0, "V_PV2"=0.0, "V_CAP2"=0.0, "V_grid2"=0.0, "V_PV3"=0.0, "V_CAP3"=0.0, "V_grid3"=0.0, "V_PV4"=0.0, "V_CAP4"=0.0, "V_grid4"=0.0, "V_grid1"=0.0, "P1"=0.0, "P2"=0.0, "P3"=0.0, "P4"=0.0}, "Status 3"=FALSE, "Status 4"=FALSE, "measurements SC"={"V_SC"=0.0, "V_CAP"=0.0, "V_grid"=0.0, "P"=0.0, "SOC"=0.0}, "Status SC"=FALSE, "Forming/Following"=FALSE, "Start forming"=FALSE, "SC references"={"Vdc"=0.0, "Pdc"=0.0}, "Start following"=FALSE}} ("PV+SC"), error in (no error)=w230) -> (value=w232:T9, error out=w231:errorcluster)  [unwired: 4 in]
      }
    }
    n77 = Bundle By Name(cluster=w194, "Data.measurements SC.SOC"="SOC") -> (w193:T9)
    n78 = local read "Stop"() -> (w207:bool)
    n79 = Select(t=w194, s="SC_include", f=w193) -> (s? t:f=w195:T9)
    n80 = local write "IN PV+SC"(w195) -> ()
  }
  n81 = while {
    tunnel: w79 -> [w246]
    tunnel: w78 -> [w257]
    shift-right: [w240] -> w82
    shift-left: w86 -> [w244]
    tunnel: w85 -> [w243]
    tunnel: [w245] -> w81
    stop <- w247 stop-if-true
    n82 = Wait (ms)(milliseconds to wait=u32 100) -> ()  [unwired: 1 out]
    n83 = local read "OUT cOPF"() -> (w251:T22)
    n84 = Flatten To JSON(anything=w251, error in (no error)=w243) -> (JSON string=w252:string, 11:w250:errorcluster)  [unwired: 1 in]
    n85 = UDP Write(address=w246, port or service name=w257, connection ID=w244, data in=w252, 8:w250) -> (error out=w241:errorcluster, 3:w242:refnum<k16>)  [unwired: 1 in]
    n86 = UDP Read(connection ID=w242, max size (548)=4000, timeout ms (25000)=500, 8:w241) -> (data out=w255:string, error out=w254:errorcluster, 3:w240:refnum<k16>)  [unwired: 2 out]
    n87 = call <vilib>:"Is Empty.vi"("JSON"=w255) -> ("Empty"=w253:bool)  [unwired: 4 in]
    n88 = Not(x=w253) -> (.not. x?=→"cOPF data":bool)
    n89 = case shown="False" w253 {
      tunnel: w254 -> [w259 w263]
      tunnel: w255 -> [_ w262]
      tunnel: [w259 w264] -> w245
      tunnel: [w258 w260] -> w239
      frame True {
        (unwired) FALSE ("Found")
        n90 = local read "IN cOPF"() -> (w258:T22)
      }
      frame False {
        n91 = Unflatten From JSON(JSON string=w262, type and defaults=T22 {"Info"={"Resource"="Zenone", "Problem"=0.0, "Timestamp"=0.0}, "Data"={"Operation_mode"="Grid connected", "solution_feasible"=0.0, "Optimal_slack"="AFE 1", "setpoints"=[], "upper_layer_grid_info"={"Frequency"=0.0, "Angle"=0.0, "Magnitude"=0.0}, "SC_soc"=0.0, "PV"={"perun"=0.0, "solarmax"=0.0, "facade"=0.0, "emul4"=0.0, "emul5"=0.0, "emul6"=0.0, "emul7"=0.0}, "P_pv_facade"=0.0}} ("IN iOPF"), error in (no error)=w263) -> (value=w260:T22, error out=w264:errorcluster)  [unwired: 4 in]
      }
    }
    n92 = Unbundle By Name(w239) -> ("Info.Timestamp"=w233:dbl, "Data.setpoints"=w238:dbl[])
    n93 = local write "IN cOPF"(w239) -> ()
    n94 = local read "Stop"() -> (w247:bool)
    n95 = To Time Stamp(1:w233) -> (0:→"time connected":timestamp)
    n96 = Index Array(array=w238, index=10) -> (element=→"P_bess_connected":dbl)
  }
  n97 = while {
    tunnel: w76 -> [w289]
    tunnel: w75 -> [w288]
    shift-right: [w273] -> w84
    shift-left: w92 -> [w278]
    tunnel: w91 -> [w275]
    tunnel: [w279] -> w83
    stop <- w282 stop-if-true
    n98 = local read "OUT iOPF"() -> (w280:T22)
    n99 = Wait (ms)(milliseconds to wait=u32 100) -> ()  [unwired: 1 out]
    n100 = Flatten To JSON(anything=w280, error in (no error)=w275) -> (JSON string=w281:string, 11:w274:errorcluster)  [unwired: 1 in]
    n101 = UDP Write(address=w288, port or service name=w289, connection ID=w278, data in=w281, 8:w274) -> (error out=w276:errorcluster, 3:w277:refnum<k16>)  [unwired: 1 in]
    n102 = UDP Read(connection ID=w277, max size (548)=4000, timeout ms (25000)=500, 8:w276) -> (data out=w272:string, error out=w286:errorcluster, 3:w273:refnum<k16>)  [unwired: 2 out]
    n103 = call <vilib>:"Is Empty.vi"("JSON"=w272) -> ("Empty"=w285:bool)  [unwired: 4 in]
    n104 = Not(x=w285) -> (.not. x?=→"iOPF data":bool)
    n105 = case shown="False" w285 {
      tunnel: w286 -> [w291 w293]
      tunnel: [w290 w296] -> w268
      tunnel: w272 -> [_ w292]
      tunnel: [w291 w295] -> w279
      frame True {
        (unwired) FALSE ("Found")
        n106 = local read "IN iOPF"() -> (w290:T22)
      }
      frame False {
        n107 = Unflatten From JSON(JSON string=w292, type and defaults=T22 {"Info"={"Resource"="Zenone", "Problem"=0.0, "Timestamp"=0.0}, "Data"={"Operation_mode"="Grid connected", "solution_feasible"=0.0, "Optimal_slack"="AFE 1", "setpoints"=[], "upper_layer_grid_info"={"Frequency"=0.0, "Angle"=0.0, "Magnitude"=0.0}, "SC_soc"=0.0, "PV"={"perun"=0.0, "solarmax"=0.0, "facade"=0.0, "emul4"=0.0, "emul5"=0.0, "emul6"=0.0, "emul7"=0.0}, "P_pv_facade"=0.0}} ("IN cOPF"), error in (no error)=w293) -> (value=w296:T22, error out=w295:errorcluster)  [unwired: 4 in]
      }
    }
    n108 = Unbundle By Name(w268) -> ("Info.Timestamp"=w266:dbl, "Data.setpoints"=w271:dbl[])
    n109 = local write "IN iOPF"(w268) -> ()
    n110 = local read "Stop"() -> (w282:bool)
    n111 = Index Array(array=w271, index=10) -> (element=→"P_bess_island":dbl)
    n112 = To Time Stamp(1:w266) -> (0:→"time island":timestamp)
  }
  n113 = while {
    tunnel: w15 -> [w304]
    tunnel: [w299] -> w14
    shift-right: [w298] -> w13
    shift-left: w16 -> [w305]
    stop <- w297 stop-if-true
    n114 = UDP Read(connection ID=w305, 8:w304) -> (data out=w302:string, error out=w300:errorcluster, 3:w298:refnum<k16>)  [unwired: 2 in, 2 out]
    n115 = call <vilib>:"Is Empty.vi"("JSON"=w302) -> ("Empty"=w303:bool)  [unwired: 4 in]
    n116 = case shown="False" w303 {
      tunnel: w302 -> [_ w312]
      tunnel: [w307 w310] -> w301
      tunnel: w300 -> [w306 w309]
      tunnel: [w306 w308] -> w299
      frame True {
        n117 = local read "IN Meteo"() -> (w307:T6)
      }
      frame False {
        n118 = Unflatten From JSON(JSON string=w312, type and defaults=T6 {"Info"={"Resource"="MeteoBox", "Problem"=FALSE, "Timestamp"=0.0}, "Data"={"GI"=0.0, "GHI"=0.0, "GVI"=0.0, "Tair"=0.0, "Tcell roof"=0.0, "Global_Total_Irr"=0.0, "Diffused_Irr"=0.0, "Tcell facade"=0.0, "PV_mpp"={"perun"=0.0, "solarmax"=0.0, "facade"=0.0, "emul4"=0.0, "emul5"=0.0, "emul6"=0.0, "emul7"=0.0}}} ("Cluster"), error in (no error)=w309) -> (value=w310:T6, error out=w308:errorcluster)  [unwired: 4 in]
      }
    }
    n119 = local write "IN Meteo"(w301) -> ()
    n120 = local read "Stop"() -> (w297:bool)
  }
  n121 = Initialize Array(FALSE, "nb instances") -> (w104:bool[])
  n122 = Initialize Array(FALSE, "nb instances") -> (w102:bool[])
  n123 = String To IP(1:w30) -> (0:w29:u32)
  n124 = String To IP(1:w34) -> (0:w35:u32)
  n125 = UDP Open(7:w35, 9:5000 ("timeout ms (25000)"), 11:w32) -> (port=w31:refnum<k16>, 0:w22:errorcluster)  [unwired: 2 in, 1 out]
  n126 = while {
    tunnel: [w319] -> w36
    tunnel: w29 -> [w329]
    tunnel: w28 -> [w328]
    tunnel: w22 -> [w323]
    shift-right: [w318] -> w21
    shift-left: w31 -> [w330]
    stop <- w326 stop-if-true
    # "Central data aquisition"
    n127 = local read "Zenone_Q"() -> (w324:dbl)
    n128 = local read "Zenone_P"() -> (w325:dbl)
    n129 = local read "setpoints"() -> (w332:dbl[])
    n130 = Wait (ms)(milliseconds to wait=u32 100) -> ()  [unwired: 1 out]
    n131 = call "Setpoint.vi"("ZENONE.Q_set [kVAr]"=w324, "ZENONE.P_set [kW]"=w325, "setpoints IN"=w332) -> ("OUT"=w313:T4)  [unwired: 8 in]
    n132 = Flatten To JSON(anything=w313) -> (JSON string=w331:string)  [unwired: 2 in, 1 out]
    n133 = case shown="True" "Send sp AC?" {
      tunnel: w331 -> [_ w357]
      tunnel: w330 -> [w350 w356]
      tunnel: w329 -> [_ w355]
      tunnel: w328 -> [_ w354]
      tunnel: [w350 w353] -> w321
      tunnel: [w349 w352] -> w320
      tunnel: w323 -> [w349 w351]
      frame False {
      }
      frame True {
        n134 = UDP Write(address=w355, port or service name=w354, connection ID=w356, data in=w357, 8:w351) -> (error out=w352:errorcluster, 3:w353:refnum<k16>)  [unwired: 1 in]
      }
    }
    n135 = UDP Read(connection ID=w321, max size (548)=2000, 8:w320) -> (data out=w316:string, error out=w317:errorcluster, 3:w318:refnum<k16>)  [unwired: 1 in, 2 out]
    n136 = call <vilib>:"Is Empty.vi"("JSON"=w316) -> ("Empty"=w315:bool)  [unwired: 4 in]
    n137 = case shown="False" w315 {
      tunnel: [w333 w340] -> w319
      tunnel: w316 -> [_ w339]
      tunnel: w317 -> [w333 w335]
      frame True {
      }
      frame False {
        n138 = call <vilib>:"Find Item.vi"("$Path or Item Name"="Facade", "JSON"=w339) -> ("<JSON>"=w337:string, "Found"=w336:bool)  [unwired: 6 in, 2 out]
        n139 = case shown="False" w336 {
          tunnel: w337 -> [_ w348]
          tunnel: w335 -> [w342 w347]
          tunnel: [w342 w346] -> w340
          tunnel: [w341 w343] -> w334
          frame False {
            n140 = local read "P_pv_facade"() -> (w341:dbl)
          }
          frame True {
            n141 = Unflatten From JSON(JSON string=w348, type and defaults=T31 {"Info"={"Resource"="Zenone", "Problem"=FALSE, "Timestamp"=0.0}, "Data"={"P"=0.0, "Q"=0.0, "Pset"=0.0, "Qset"=0.0}} ("Cluster"), error in (no error)=w347) -> (value=w344:T31, error out=w346:errorcluster)  [unwired: 4 in]
            n142 = Unbundle By Name(w344) -> ("Data.P"=w343:dbl)
          }
        }
        n143 = local write "P_pv_facade"(w334) -> ()
      }
    }
    n144 = local read "Stop"() -> (w326:bool)
  }
  n145 = node-c288() -> (w99:T34)  [unwired: 4 in]
  n146 = timed-loop {
    shift-right: [w377] -> _
    shift-left: w104 -> [w378]
    shift-right: [w375] -> _
    shift-left: w102 -> [w376]
    tunnel: "nb instances" -> [w374]
    shift-right: [w367] -> _
    shift-left: State_Machine."Grid connected" ("State") -> [w368]
    timing: w99 -> [_]
    timing-out: [_] -> w98
    stop <- "Stop" stop-if-true
    # "State Machine While Loop"
    n147 = node-c288() -> ()  [unwired: 1 in, 1 out]
    n148 = case "State Machine Case Structure" shown="\"Island\"" w368 {
      tunnel: "IN synchro" -> [w405 w495 w599 w716]
      tunnel: "IN AFE" -> [w404 w496 w600 w715]
      tunnel: "IN cOPF" -> [w403 w497 w601 w714]
      tunnel: "IN iOPF" -> [w402 w498 w602 w713]
      tunnel: "slack" -> [w401 w489 w603 w712]
      tunnel: w378 -> [w400 w494 w598 w711]
      tunnel: [w400 w493 w598 w711] -> w377
      tunnel: w376 -> [w399 w492 w597 w710]
      tunnel: [w399 w491 w597 w710] -> w375
      tunnel: w374 -> [_ w490 _ _]
      tunnel: [w395 w481 w593 w706] -> w373
      tunnel: [w397 w483 w594 w707] -> w372
      tunnel: [w396 w482 w595 w708] -> w371
      tunnel: [w398 w484 w596 w709] -> w370
      tunnel: [w383 w470 w581 w694] -> w367
      tunnel: "IN PV+SC" -> [w389 w474 w586 w699]
      tunnel: [w388 w471 w583 w696] -> w360
      tunnel: "IN Meteo" -> [w382 w467 w579 w690]
      tunnel: "SCADA" -> [_ w464 w577 _]
      frame "Grid connected", Default {
        # "Grid connected - Display a dialog box with a message specific to State 1, then go back to the Wait for Event state."
        n149 = flat-sequence {
          tunnel: w405 -> [w424]
          tunnel: w404 -> [w425]
          tunnel: w403 -> [w423]
          tunnel: w402 -> [w422]
          tunnel: w401 -> [w426]
          tunnel: [w425] -> w394
          tunnel: [w424] -> w393
          tunnel: [w423] -> w392
          tunnel: [w422] -> w391
          tunnel: [w413] -> w390
          tunnel: w389 -> [w414]
          tunnel: [w421] -> w387
          tunnel: [w414] -> w386
          tunnel: [w413] -> w385
          tunnel: w382 -> [w409]
          tunnel: [w408] -> w381
          tunnel: w394 -> [w457]
          tunnel: w393 -> [w456]
          tunnel: w392 -> [w455]
          tunnel: w391 -> [w454]
          tunnel: w390 -> [w452]
          tunnel: w387 -> [w451]
          tunnel: w386 -> [w449]
          tunnel: w385 -> [w446]
          tunnel: [w461] -> w398
          tunnel: [w460] -> w397
          tunnel: [w459] -> w396
          tunnel: [w458] -> w395
          tunnel: [w450] -> w388
          tunnel: w381 -> [w438]
          frame #0 {
            # "from slack selection"
            # "from island OPF"
            # "from connected OPF"
            # "from resource"
            # "from synchrocheck"
            n150 = Unbundle By Name(w414) -> ("Data.Forming/Following"=→"forming SC?":bool, "Data.measurements SC.SOC"=w410:dbl)
            n151 = Unbundle By Name(w424) -> ("Data.Synchronised?"=→"synchronised?":bool, "Data.V_UpStream"=w412:T28, "Data.V_Downstream"=w411:T28)
            n152 = Unbundle By Name(w409) -> ("Data.PV_mpp"=w408:T38)
            n153 = Unbundle By Name(w425) -> ("Data.Forming/Following"=w432:bool[])
            n154 = Unbundle By Name(w423) -> ("Data.solution_feasible"=w418:dbl, "Data.setpoints"=w413:dbl[])
            n155 = Unbundle By Name(w422) -> ("Data.solution_feasible"=w420:dbl)
            n156 = Unbundle By Name(w426) -> ("Data.Optimal slack"=→"optimal_slack":string, "Data.Time-To-Live"=w416:dbl)
            n157 = local write "to grid connection"(TRUE ("to grid connection")) -> ()
            n158 = local write "to prepare for island"(FALSE ("to prepare for island")) -> ()
            n159 = local write "to island"(FALSE ("to island")) -> ()
            n160 = local write "to prepare for grid connection"(FALSE ("to prepare for grid connection")) -> ()
            n161 = Not Equal To 0?(x=w418) -> (x != 0?=→"cOPF valid?":bool)
            n162 = Not Equal To 0?(x=w420) -> (x != 0?=→"iOPF valid":bool)
            n163 = local write "Time-To-Live (minutes)"(w416) -> ()
            n164 = local write "setpoints"(w413) -> ()
            n165 = Or Array Elements(Boolean array=w432) -> (logical OR=→"forming AFE?":bool)
            n166 = local write "SC_soc"(w410) -> ()
            n167 = call "up_grid_data.vi"("Data.V_Downstream"=w411, "Data.V_UpStream"=w412) -> ("upper layer grid info"=w421:T37)  [unwired: 5 in, 4 out]
          }
          frame #1 {
            # "send to island OPF"
            # "send to resource"
            # "send to connected OPF"
            # "send to synchrocheck"
            n168 = local read "P_pv_facade"() -> (w435:dbl)
            n169 = local read "SC_soc"() -> (w440:dbl)
            n170 = local read "SC_soc"() -> (w439:dbl)
            n171 = call "distribute_setpoints.vi"("setpoints"=w452, "upper layer grid info"=w451) -> ("references"=w453:T21)  [unwired: 9 in]
            n172 = call "distribute_setpoints_DC.vi"("setpoints"=w446) -> ("reference_DC"=w447:T14)  [unwired: 10 in]
            n173 = Bundle By Name(cluster=w455, "Data.Operation_mode"="Grid connected" ("Operation_mode"), "Data.upper_layer_grid_info"=w451, "Data.SC_soc"=w440, "Data.P_pv_facade"=w435, "Data.PV"=w438) -> (w459:T22)
            n174 = Bundle By Name(cluster=w454, "Data.Operation_mode"="Grid connected" ("Operation_mode"), "Data.upper_layer_grid_info"=w451, "Data.SC_soc"=w439, "Data.P_pv_facade"=w435, "Data.PV"=w438) -> (w461:T22)
            n175 = Bundle By Name(cluster=w449, "Data.Start following"=TRUE, "Data.Start forming"=FALSE, "Data.SC references"=w447) -> (w450:T9)
            n176 = Bundle By Name(cluster=w456, "Data.close/open relay"=TRUE, "Data.Operation mode"="Grid connected" ("Operation_mode")) -> (w458:T25)
            n177 = Bundle By Name(cluster=w457, "Data.Start forming 2"=FALSE, "Data.Start following 2"=TRUE, "Data.Start following 1"=TRUE, "Data.Start forming 1"=FALSE, "Data.references"=w453) -> (w460:T18)
          }
        }
        n178 = case shown="True" "to prepare for island" {
          tunnel: [State_Machine."Grid connected" ("State") State_Machine."Prepare for island" ("State")] -> w383
          frame False {
          }
          frame True {
          }
        }
      }
      frame "Prepare for island" {
        n179 = flat-sequence {
          tunnel: w498 -> [w525]
          tunnel: w497 -> [w524]
          tunnel: w496 -> [w522]
          tunnel: w495 -> [w523]
          tunnel: w494 -> [w536]
          tunnel: w492 -> [w534]
          tunnel: w490 -> [w530]
          tunnel: w489 -> [w529]
          tunnel: [w535] -> w488
          tunnel: [w533] -> w487
          tunnel: [w532] -> w486
          tunnel: [w531] -> w485
          tunnel: [w525] -> w480
          tunnel: [w524] -> w479
          tunnel: [w523] -> w478
          tunnel: [w522] -> w477
          tunnel: [w514] -> w476
          tunnel: [w521] -> w475
          tunnel: w474 -> [w515]
          tunnel: [w515] -> w473
          tunnel: [w514] -> w472
          tunnel: w467 -> [w506]
          tunnel: [w505] -> w466
          tunnel: w464 -> [_]
          tunnel: w488 -> [w572]
          tunnel: w487 -> [w571]
          tunnel: w486 -> [w551]
          tunnel: w485 -> [w552]
          tunnel: w480 -> [w562]
          tunnel: w479 -> [w561]
          tunnel: w478 -> [w560]
          tunnel: w477 -> [w559]
          tunnel: w476 -> [w557]
          tunnel: w475 -> [w546]
          tunnel: w473 -> [w556]
          tunnel: w472 -> [w553]
          tunnel: [w572] -> w493
          tunnel: [w571] -> w491
          tunnel: [w566] -> w484
          tunnel: [w565] -> w483
          tunnel: [w564] -> w482
          tunnel: [w563] -> w481
          tunnel: [w555] -> w471
          tunnel: [w552] -> w469
          tunnel: [w551] -> w468
          tunnel: w466 -> [w541]
          frame #0 {
            # "from slack selection"
            # "from island OPF"
            # "from connected OPF"
            # "from resource"
            # "from synchrocheck"
            n180 = Unbundle By Name(w506) -> ("Data.PV_mpp"=w505:T38)
            n181 = Unbundle By Name(w515) -> ("Data.Forming/Following"=w516:bool, "Data.measurements SC.SOC"=w507:dbl)
            n182 = Unbundle By Name(w524) -> ("Data.solution_feasible"=w518:dbl, "Data.setpoints"=w514:dbl[])
            n183 = Unbundle By Name(w522) -> ("Data.Forming/Following"=w537:bool[])
            n184 = Unbundle By Name(w525) -> ("Data.solution_feasible"=w519:dbl)
            n185 = Unbundle By Name(w529) -> ("Data.Time-To-Live"=w528:dbl)
            n186 = Unbundle By Name(w523) -> ("Data.Synchronised?"=w527:bool, "Data.V_UpStream"=w509:T28, "Data.V_Downstream"=w508:T28)
            n187 = local write "to grid connection"(FALSE ("to grid connection")) -> ()
            n188 = local write "to prepare for island"(TRUE ("to prepare for island")) -> ()
            n189 = local write "to island"(FALSE ("to island")) -> ()
            n190 = local write "to prepare for grid connection"(FALSE ("to prepare for grid connection")) -> ()
            n191 = local write "synchronised?"(w527) -> ()
            n192 = Or Array Elements(Boolean array=w537) -> (logical OR=w526:bool)
            n193 = local write "setpoints"(w514) -> ()
            n194 = local write "Time-To-Live (minutes)"(w528) -> ()
            n195 = local write "forming SC?"(w516) -> ()
            n196 = local write "SC_soc"(w507) -> ()
            n197 = Not Equal To 0?(x=w518) -> (x != 0?=w517:bool)
            n198 = Not Equal To 0?(x=w519) -> (x != 0?=w520:bool)
            n199 = local write "forming AFE?"(w526) -> ()
            n200 = call "check multiple instances.vi"("nb instances"=w530, "array elements in"=w536, "new element"=w517) -> ("array elements out"=w535:bool[], "out"=w531:bool)  [unwired: 7 in]
            n201 = local write "cOPF valid?"(w517) -> ()
            n202 = call "check multiple instances.vi"("nb instances"=w530, "array elements in"=w534, "new element"=w520) -> ("array elements out"=w533:bool[], "out"=w532:bool)  [unwired: 7 in]
            n203 = local write "iOPF valid"(w520) -> ()
            n204 = call "up_grid_data.vi"("Data.V_Downstream"=w508, "Data.V_UpStream"=w509) -> ("upper layer grid info"=w521:T37)  [unwired: 5 in, 4 out]
          }
          frame #1 {
            # "send to island OPF"
            # "send to resource"
            # "send to connected OPF"
            # "send to synchrocheck"
            n205 = local read "P_pv_facade"() -> (w538:dbl)
            n206 = local read "optimal_slack"() -> (w569:string)
            n207 = local read "optimal_slack"() -> (w570:string)
            n208 = call "distribute_setpoints_DC.vi"("setpoints"=w553) -> ("reference_DC"=w545:T14)  [unwired: 10 in]
            n209 = call "distribute_setpoints.vi"("setpoints"=w557, "upper layer grid info"=w546) -> ("references"=w558:T21)  [unwired: 9 in]
            n210 = local read "SC_soc"() -> (w543:dbl)
            n211 = local read "SC_soc"() -> (w542:dbl)
            n212 = Bundle By Name(cluster=w561, "Data.Operation_mode"="Prepare Island" ("Operation_mode"), "Data.Optimal_slack"=w569, "Data.upper_layer_grid_info"=w546, "Data.SC_soc"=w543, "Data.P_pv_facade"=w538, "Data.PV"=w541) -> (w564:T22)
            n213 = Bundle By Name(cluster=w562, "Data.Operation_mode"="Prepare Island" ("Operation_mode"), "Data.Optimal_slack"=w570, "Data.upper_layer_grid_info"=w546, "Data.SC_soc"=w542, "Data.P_pv_facade"=w538, "Data.PV"=w541) -> (w566:T22)
            n214 = Bundle By Name(cluster=w560, "Data.close/open relay"=TRUE, "Data.Operation mode"="Prepare Island" ("Operation_mode")) -> (w563:T25)
            n215 = Bundle By Name(cluster=w559, "Data.Start forming 2"=FALSE, "Data.Start following 2"=TRUE, "Data.Start following 1"=TRUE, "Data.Start forming 1"=FALSE, "Data.references"=w558) -> (w565:T18)
            n216 = Bundle By Name(cluster=w556, "Data.Start following"=TRUE, "Data.Start forming"=FALSE, "Data.SC references"=w545) -> (w555:T9)
          }
        }
        n217 = disable-structure shown="Disabled" {
          disable-tunnel: [w502 _] -> _
          disable-tunnel: "to island" -> [w501 _]
          disable-tunnel: w469 -> [w500 _]
          disable-tunnel: w468 -> [w499 _]
          frame Disabled {
            n218 = Compound Arithmetic op=AND(w500, w499, w501) -> (w502:bool)
          }
          frame Enabled {
          }
        }
        n219 = case shown="False" "to island" {
          tunnel: [State_Machine."Prepare for island" ("State") State_Machine."Island" ("State")] -> w470
          frame False {
          }
          frame True {
            # "only go to next state if OPFs are feasible for 7 timesteps"
          }
        }
      }
      frame "Island" {
        # "Island - Display a dialog box with a message specific to State 3, then go back to the Wait for Event state."
        n220 = flat-sequence {
          tunnel: w603 -> [w640]
          tunnel: w602 -> [w632]
          tunnel: w601 -> [w631]
          tunnel: w600 -> [w630]
          tunnel: w599 -> [w629]
          tunnel: [w632] -> w592
          tunnel: [w631] -> w591
          tunnel: [w630] -> w590
          tunnel: [w629] -> w589
          tunnel: [w622] -> w588
          tunnel: [w614] -> w587
          tunnel: w586 -> [w623]
          tunnel: [w623] -> w585
          tunnel: [w622] -> w584
          tunnel: [w619] -> w580
          tunnel: w579 -> [w617]
          tunnel: [w616] -> w578
          tunnel: w577 -> [w615]
          tunnel: [w613] -> w576
          tunnel: [w610] -> w575
          tunnel: ["PI on V"] -> w574
          tunnel: [w607] -> w573
          tunnel: w592 -> [w659]
          tunnel: w591 -> [w678]
          tunnel: w590 -> [w677]
          tunnel: w589 -> [w676]
          tunnel: w588 -> [w674]
          tunnel: w587 -> [w653]
          tunnel: w585 -> [w673]
          tunnel: w584 -> [w670]
          tunnel: [w682] -> w596
          tunnel: [w681] -> w595
          tunnel: [w680] -> w594
          tunnel: [w679] -> w593
          tunnel: [w672] -> w583
          tunnel: w580 -> [_]
          tunnel: w578 -> [w658]
          tunnel: w576 -> [w651]
          tunnel: w575 -> [w642]
          tunnel: w574 -> [w649]
          tunnel: w573 -> [w643]
          frame #0 {
            # "from slack selection"
            # "from island OPF"
            # "from connected OPF"
            # "from resource"
            # "from synchrocheck"
            n221 = Unbundle By Name(w623) -> ("Data.Forming/Following"=w624:bool, "Data.measurements SC.SOC"=w618:dbl)
            n222 = Unbundle By Name(w632) -> ("Data.solution_feasible"=w628:dbl, "Data.setpoints"=w622:dbl[], "Data.upper_layer_grid_info"=w619:T37)
            n223 = Unbundle By Name(w630) -> ("Data.Forming/Following"=w641:bool[])
            n224 = Unbundle By Name(w631) -> ("Data.solution_feasible"=w627:dbl)
            n225 = Unbundle By Name(w629) -> ("Data.Synchronised?"=w634:bool, "Data.V_UpStream"=w621:T28, "Data.V_Downstream"=w620:T28)
            n226 = Unbundle By Name(w640) -> ("Data.Time-To-Live"=w639:dbl)
            n227 = Unbundle By Name(w615) -> ("Data.Voltage mag"=w612:dbl[])  [unwired: 1 out]
            n228 = Unbundle By Name(w617) -> ("Data.PV_mpp"=w616:T38)
            n229 = local write "to grid connection"(FALSE ("to grid connection")) -> ()
            n230 = local write "to prepare for island"(FALSE ("to prepare for island")) -> ()
            n231 = local write "to island"(TRUE ("to island")) -> ()
            n232 = local write "to prepare for grid connection"(FALSE ("to prepare for grid connection")) -> ()
            n233 = local write "Time-To-Live (minutes)"(w639) -> ()
            n234 = local write "synchronised?"(w634) -> ()
            n235 = Not Equal To 0?(x=w627) -> (x != 0?=w626:bool)
            n236 = local write "setpoints"(w622) -> ()
            n237 = Not Equal To 0?(x=w628) -> (x != 0?=w625:bool)
            n238 = Or Array Elements(Boolean array=w641) -> (logical OR=w633:bool)
            n239 = local write "forming SC?"(w624) -> ()
            n240 = local write "SC_soc"(w618) -> ()
            n241 = local write "forming AFE?"(w633) -> ()
            n242 = local write "cOPF valid?"(w626) -> ()
            n243 = Index Array(array=w612, index #1=18 ("index"), index #2=14 ("index")) -> (element #1=w610:dbl, element #2=w607:dbl)
            n244 = local write "iOPF valid"(w625) -> ()
            n245 = call "up_grid_data.vi"("Data.V_Downstream"=w620, "Data.V_UpStream"=w621) -> ("upper layer grid info"=w614:T37)  [unwired: 5 in, 4 out]
            n246 = Unbundle By Name(w614) -> ("Magnitude"=w613:dbl)
          }
          frame #1 {
            (unwired) 50.0 ("Frequency")
            # "send to island OPF"
            # "send to connected OPF"
            # "send to resource"
            # "send to synchrocheck"
            n247 = Unbundle(w653) -> ("Frequency"=w652:dbl)  [unwired: 2 out]
            n248 = call <userlib>:"Boolean Trigger__ogtk.vi"("Boolean Input"=w649) -> ("Rising Edge"=w650:bool)  [unwired: 1 in, 1 out]
            n249 = local read "optimal_slack"() -> (w686:string)
            n250 = local read "P_pv_facade"() -> (w654:dbl)
            n251 = call "PID2_2V.vi"("reinitialize? (F)"=w650, "V_afe"=w642, "V_up"=w651) -> ("output"=w645:dbl)  [unwired: 8 in]
            n252 = local read "optimal_slack"() -> (w685:string)
            n253 = call "distribute_setpoints_DC.vi"("setpoints"=w670) -> ("reference_DC"=w663:T14)  [unwired: 10 in]
            n254 = Select(t=w645, s=w649, f=w643) -> (s? t:f=w648:dbl)
            "V_control" <- w648
            n255 = Bundle(cluster=T37 {"Frequency"=0.0, "Angle"=0.0, "Magnitude"=0.0} ("upper layer grid info"), "Frequency"=w652, "Angle"=0.0, "Magnitude"=w648) -> (w666:T37)
            n256 = local read "SC_soc"() -> (w660:dbl)
            n257 = local read "SC_soc"() -> (w661:dbl)
            n258 = call "distribute_setpoints.vi"("setpoints"=w674, "upper layer grid info"=w666) -> ("references"=w675:T21)  [unwired: 9 in]
            n259 = Bundle(cluster=cluster{dbl, "ROCOF [Hz/s]":dbl} {229.99881816350032, "ROCOF [Hz/s]"=229.99881816350032} ("Direct sequence phase difference"), w645, "ROCOF [Hz/s]"=0.0) -> (→"V control":cluster{dbl, "ROCOF [Hz/s]":dbl})
            n260 = Bundle By Name(cluster=w678, "Data.Operation_mode"="Island" ("Operation_mode"), "Data.Optimal_slack"=w685, "Data.upper_layer_grid_info"=w653, "Data.SC_soc"=w661, "Data.P_pv_facade"=w654, "Data.PV"=w658) -> (w681:T22)
            n261 = Bundle By Name(cluster=w659, "Data.Operation_mode"="Island" ("Operation_mode"), "Data.Optimal_slack"=w686, "Data.upper_layer_grid_info"=w653, "Data.SC_soc"=w660, "Data.P_pv_facade"=w654, "Data.PV"=w658) -> (w682:T22)
            n262 = Bundle By Name(cluster=w673, "Data.Start following"=FALSE, "Data.Start forming"=TRUE, "Data.SC references"=w663) -> (w672:T9)
            n263 = Bundle By Name(cluster=w676, "Data.close/open relay"=FALSE, "Data.Operation mode"="Island" ("Operation_mode")) -> (w679:T25)
            n264 = Bundle By Name(cluster=w677, "Data.Start forming 2"=FALSE, "Data.Start following 2"=TRUE, "Data.Start following 1"=FALSE, "Data.Start forming 1"=TRUE, "Data.references"=w675) -> (w680:T18)
            "V_upstream" <- w651
            "V_afe" <- w642
          }
        }
        n265 = case shown="True" "to prepare for grid connection" {
          tunnel: [State_Machine."Island" ("State") State_Machine."Prepare for connection" ("State")] -> w581
          frame False {
          }
          frame True {
            # "only go to next state if OPFs are feasible\n for 7 timesteps"
            n266 = local write "delta angle"(0.0 ("delta angle")) -> ()
          }
        }
      }
      frame "Prepare for connection" {
        # "prepare for connection - Display a dialog box with a message specific to State 3, then go back to the Wait for Event state."
        n267 = flat-sequence {
          tunnel: w716 -> [w735]
          tunnel: w715 -> [w736]
          tunnel: w714 -> [w737]
          tunnel: w713 -> [w738]
          tunnel: w712 -> [w746]
          tunnel: [w738] -> w705
          tunnel: [w737] -> w704
          tunnel: [w736] -> w703
          tunnel: [w735] -> w702
          tunnel: [w727] -> w701
          tunnel: [w734] -> w700
          tunnel: w699 -> [w728]
          tunnel: [w728] -> w698
          tunnel: [w727] -> w697
          tunnel: [w724] -> w693
          tunnel: [w719] -> w692
          tunnel: [w720] -> w691
          tunnel: w690 -> [w722]
          tunnel: [w721] -> w689
          tunnel: w705 -> [w780]
          tunnel: w704 -> [w779]
          tunnel: w703 -> [w778]
          tunnel: w702 -> [w777]
          tunnel: w701 -> [w775]
          tunnel: w700 -> [w764]
          tunnel: w698 -> [w774]
          tunnel: w697 -> [w770]
          tunnel: [w784] -> w709
          tunnel: [w783] -> w708
          tunnel: [w782] -> w707
          tunnel: [w781] -> w706
          tunnel: [w773] -> w696
          tunnel: w693 -> [_]
          tunnel: w692 -> [w759]
          tunnel: w691 -> [w758]
          tunnel: w689 -> [w754]
          frame #0 {
            # "from slack selection"
            # "from island OPF"
            # "from connected OPF"
            # "from resource"
            # "from synchrocheck"
            n268 = Unbundle By Name(w722) -> ("Data.PV_mpp"=w721:T38)
            n269 = Unbundle By Name(w728) -> ("Data.Forming/Following"=w729:bool, "Data.measurements SC.SOC"=w723:dbl)
            n270 = Unbundle By Name(w738) -> ("Data.solution_feasible"=w733:dbl, "Data.setpoints"=w727:dbl[], "Data.upper_layer_grid_info"=w724:T37)
            n271 = Unbundle By Name(w736) -> ("Data.Forming/Following"=w747:bool[])
            n272 = Unbundle By Name(w735) -> ("Data.Synchronised?"=w740:bool, "Data.V_UpStream"=w726:T28, "Data.V_Downstream"=w725:T28)
            n273 = Unbundle By Name(w737) -> ("Data.solution_feasible"=w731:dbl)  [unwired: 1 out]
            n274 = Unbundle By Name(w746) -> ("Data.Time-To-Live"=w745:dbl)
            n275 = local write "to grid connection"(FALSE ("to grid connection")) -> ()
            n276 = local write "to prepare for island"(FALSE ("to prepare for island")) -> ()
            n277 = local write "to island"(FALSE ("to island")) -> ()
            n278 = local write "to prepare for grid connection"(TRUE ("to prepare for grid connection")) -> ()
            n279 = local write "Time-To-Live (minutes)"(w745) -> ()
            n280 = Not Equal To 0?(x=w731) -> (x != 0?=w730:bool)
            n281 = Not Equal To 0?(x=w733) -> (x != 0?=w732:bool)
            n282 = local write "synchronised?"(w740) -> ()
            n283 = Or Array Elements(Boolean array=w747) -> (logical OR=w739:bool)
            n284 = local write "forming SC?"(w729) -> ()
            n285 = local write "setpoints"(w727) -> ()
            n286 = local write "SC_soc"(w723) -> ()
            n287 = local write "cOPF valid?"(w730) -> ()
            n288 = local write "iOPF valid"(w732) -> ()
            n289 = local write "forming AFE?"(w739) -> ()
            n290 = call "up_grid_data_prepareConnection.vi"("Data.V_Downstream"=w725, "Data.V_UpStream"=w726) -> ("upper layer grid info"=w734:T37, "DOWN_Angle_unwrap"=w720:dbl, "UP_Angle_unwrap"=w719:dbl)  [unwired: 5 in, 2 out]
          }
          frame #1 {
            # "send to island OPF"
            # "send to connected OPF"
            # "send to resource"
            # "send to synchrocheck"
            n291 = Subtract(x=w759, y=w758) -> (x-y=→"delta angle":dbl)
            n292 = Unbundle(w764) -> ("Magnitude"=w753:dbl)  [unwired: 2 out]
            n293 = call "PID2.vi"("input"=w758, "setpoint"=w759) -> ("output"=w761:dbl)  [unwired: 9 in]
            n294 = local read "P_pv_facade"() -> (w748:dbl)
            n295 = local read "optimal_slack"() -> (w787:string)
            n296 = local read "optimal_slack"() -> (w788:string)
            n297 = Add(x=w753, y="bias magnitude") -> (x+y=w752:dbl)
            n298 = local read "SC_soc"() -> (w755:dbl)
            n299 = Bundle(cluster=T37 {"Frequency"=0.0, "Angle"=0.0, "Magnitude"=0.0} ("upper layer grid info"), "Frequency"=w761, "Angle"=0.0, "Magnitude"=w752) -> (w765:T37)
            n300 = local read "SC_soc"() -> (w756:dbl)
            n301 = call "distribute_setpoints_DC.vi"("setpoints"=w770) -> ("reference_DC"=w771:T14)  [unwired: 10 in]
            n302 = call "distribute_setpoints.vi"("setpoints"=w775, "upper layer grid info"=w765) -> ("references"=w776:T21)  [unwired: 9 in]
            n303 = Bundle By Name(cluster=w779, "Data.Operation_mode"="Prepare for connection" ("Operation_mode"), "Data.Optimal_slack"=w787, "Data.upper_layer_grid_info"=w764, "Data.SC_soc"=w755, "Data.P_pv_facade"=w748, "Data.PV"=w754) -> (w783:T22)
            n304 = Bundle By Name(cluster=w780, "Data.Operation_mode"="Prepare for connection" ("Operation_mode"), "Data.Optimal_slack"=w788, "Data.upper_layer_grid_info"=w764, "Data.SC_soc"=w756, "Data.P_pv_facade"=w748, "Data.PV"=w754) -> (w784:T22)
            n305 = Bundle By Name(cluster=w774, "Data.Start following"=FALSE, "Data.Start forming"=TRUE, "Data.SC references"=w771) -> (w773:T9)
            n306 = Bundle By Name(cluster=w777, "Data.close/open relay"=FALSE, "Data.Operation mode"="Prepare for connection" ("Operation_mode")) -> (w781:T25)
            n307 = Bundle By Name(cluster=w778, "Data.Start forming 2"=FALSE, "Data.Start following 2"=TRUE, "Data.Start following 1"=FALSE, "Data.Start forming 1"=TRUE, "Data.references"=w776) -> (w782:T18)
          }
        }
        n308 = local read "synchronised?"() -> (w687:bool)
        n309 = And(x="to grid connection", y=w687) -> (x .and. y?=w688:bool)
        n310 = case shown="True" w688 {
          tunnel: [State_Machine."Prepare for connection" ("State") State_Machine."Grid connected" ("State")] -> w694
          frame False {
          }
          frame True {
            # "only go to next state if OPFs are feasible\n for 7 timesteps"
          }
        }
      }
    }
    "OUT Synchro" <- w373
    "OUT AFE" <- w372
    "OUT cOPF" <- w371
    "OUT iOPF" <- w370
    "OUT PV+SC" <- w360
    n311 = node-c288() -> ()  [unwired: 1 in, 1 out]
  }
  n312 = call-poly <vilib>:"Read Delimited Spreadsheet.vi"("file path (dialog if empty)"=path "C:/Users/admin/Documents/git-clones/acdc_centralized_controller2/Data/Zenone_profile.csv", "format (%.3f)"="%.3f", "delimiter (\\t)"=" " ("delimiter (\\t)")) -> ("all rows"=w25:dbl[][])  [unwired: 7 in, 5 out]
  n313 = UDP Close(connection ID=w2, 8:w1) -> ()  [unwired: 2 out]
  n314 = UDP Close(connection ID=w13, 8:w14) -> ()  [unwired: 2 out]
  n315 = Matrix Size(0:w25) -> (1:w12:i32)  [unwired: 1 out]
  n316 = UDP Close(connection ID=w21, 8:w36) -> ()  [unwired: 2 out]
  n317 = while {
    shift-right: [w801] -> _
    shift-left: 0 ("number of rows") -> [w799]
    tunnel: w25 -> [w794]
    tunnel: w12 -> [w795]
    stop <- w802 stop-if-true
    n318 = Quotient & Remainder(x=w799, y=w795) -> (x-y*floor(x/y)=w798:i32)  [unwired: 1 out]
    n319 = Index Array(array=w794, index (row)=w798) -> (element=w792:dbl[])  [unwired: 1 in]
    n320 = Multiply(x=0.66 ("Numeric"), y=w792) -> (x*y=w793:dbl[])
    n321 = Index Array(array=w793) -> ()  [unwired: 2 in, 2 out]
    n322 = Absolute Value(x=3.0 ("element")) -> (abs(x)=→"Zenone_Q":dbl)
    n323 = Absolute Value(x=6.0 ("element")) -> (abs(x)=→"Zenone_P":dbl)
    n324 = local read "Stop"() -> (w802:bool)
    n325 = Increment(x=w798) -> (x+1=w801:i32)
    n326 = Wait (ms)(milliseconds to wait=u32 1000) -> ()  [unwired: 1 out]
  }
  n327 = UDP Close(connection ID=w43, 8:w42) -> ()  [unwired: 2 out]
  n328 = UDP Close(connection ID=w84, 8:w83) -> ()  [unwired: 2 out]
  n329 = UDP Close(connection ID=w82, 8:w81) -> ()  [unwired: 2 out]
  n330 = UDP Close(connection ID=w47, 8:w46) -> ()  [unwired: 2 out]
  n331 = UDP Close(connection ID=w45, 8:w44) -> ()  [unwired: 2 out]
  n332 = node-c288(w98) -> ()  [unwired: 1 out]
